vi "Station Detail Main.vi"(8 "error in (no error)":errorcluster, 11 "AI in":refnum<class "AI.lvclass">) -> (0 "error out":errorcluster, 2 "Station Out":T1=enum."ImformOut", 3 "AI out":refnum<class "AI.lvclass">)   [LabVIEW 2019, in "AI.lvclass"]
uses:
  AI.lvclass
  Ctrl/Station Action.ctl
  Ctrl/ProjectStepSelect.ctl
  Ctrl/StationCmdSelect.ctl
  Ctrl/Auto Inspection Station Name2.ctl
  Ctrl/Auto Inspection Data Name.ctl
  Ctrl/S2 Station IO.ctl
  Ctrl/MeasureDisplayTab.ctl
  Ctrl/Table Save.ctl
  Ctrl/S2 Station Input.ctl
  Global/Process Global.vi
  LLB/Commonly VI/Main Glb.vi
  LineScan/LineScan.lvclass
  LLB/Commonly VI.lvlib
panel:
  out "ToolStringOut_P1_2 2":string
  out "P1 Receive 2":string[](array[string])
  out "ToolStringOut_P1 2":string
  out "Program receive 2":string
  out "Initial receive 2":string
  out "Array":string[](array[string])
  out "Blue Scan receive":string
  out "S1 ChkSum":string
  out "S1 ToolStringOut":string
  out "ToolStringOut_P1_2":string
  out "P1 Receive":string[](array[string])
  out "ToolStringOut_P1":string
  out "ToolStringOut_Init":string
  out "Initial_ChkSum":string
  in  "Table Control":string[][](table)=[["PCBA BARCODE", ""], ["硬體(Tool初始化)", ""], ["company(Tool初始化)", ""], ["耗電流 uA(電流表)", "T"], ["電池負載電壓", "T"], ["晶片ID(Tool FORMAT)", "F"], ["雷雕ID(TOOl scan、藍芽接收器)", "S"], ["Format(Tool FORMAT)", "F"], ["Programe(Tool Programe)", "P"]]
  out "Numeric":dbl
  out "subarray":string[](array[string])
  out "T2 buffer":string
  out "T2 μA":dbl format="%#_6f"
  out "T1 buffer":string
  out "T1 μA":dbl format="%#_6f"
  out "S2 receive":string
  out "Blue Scan2 receive":string
  out "S1 receive":string
  out "Program receive":string
  out "format receive":string
  out "Initial receive":string
  out "present":i32
  out "Retry":i32
  out "Act Step":i32
  out "retry次數":string[](array[string])
  out "CurrentCmd":string
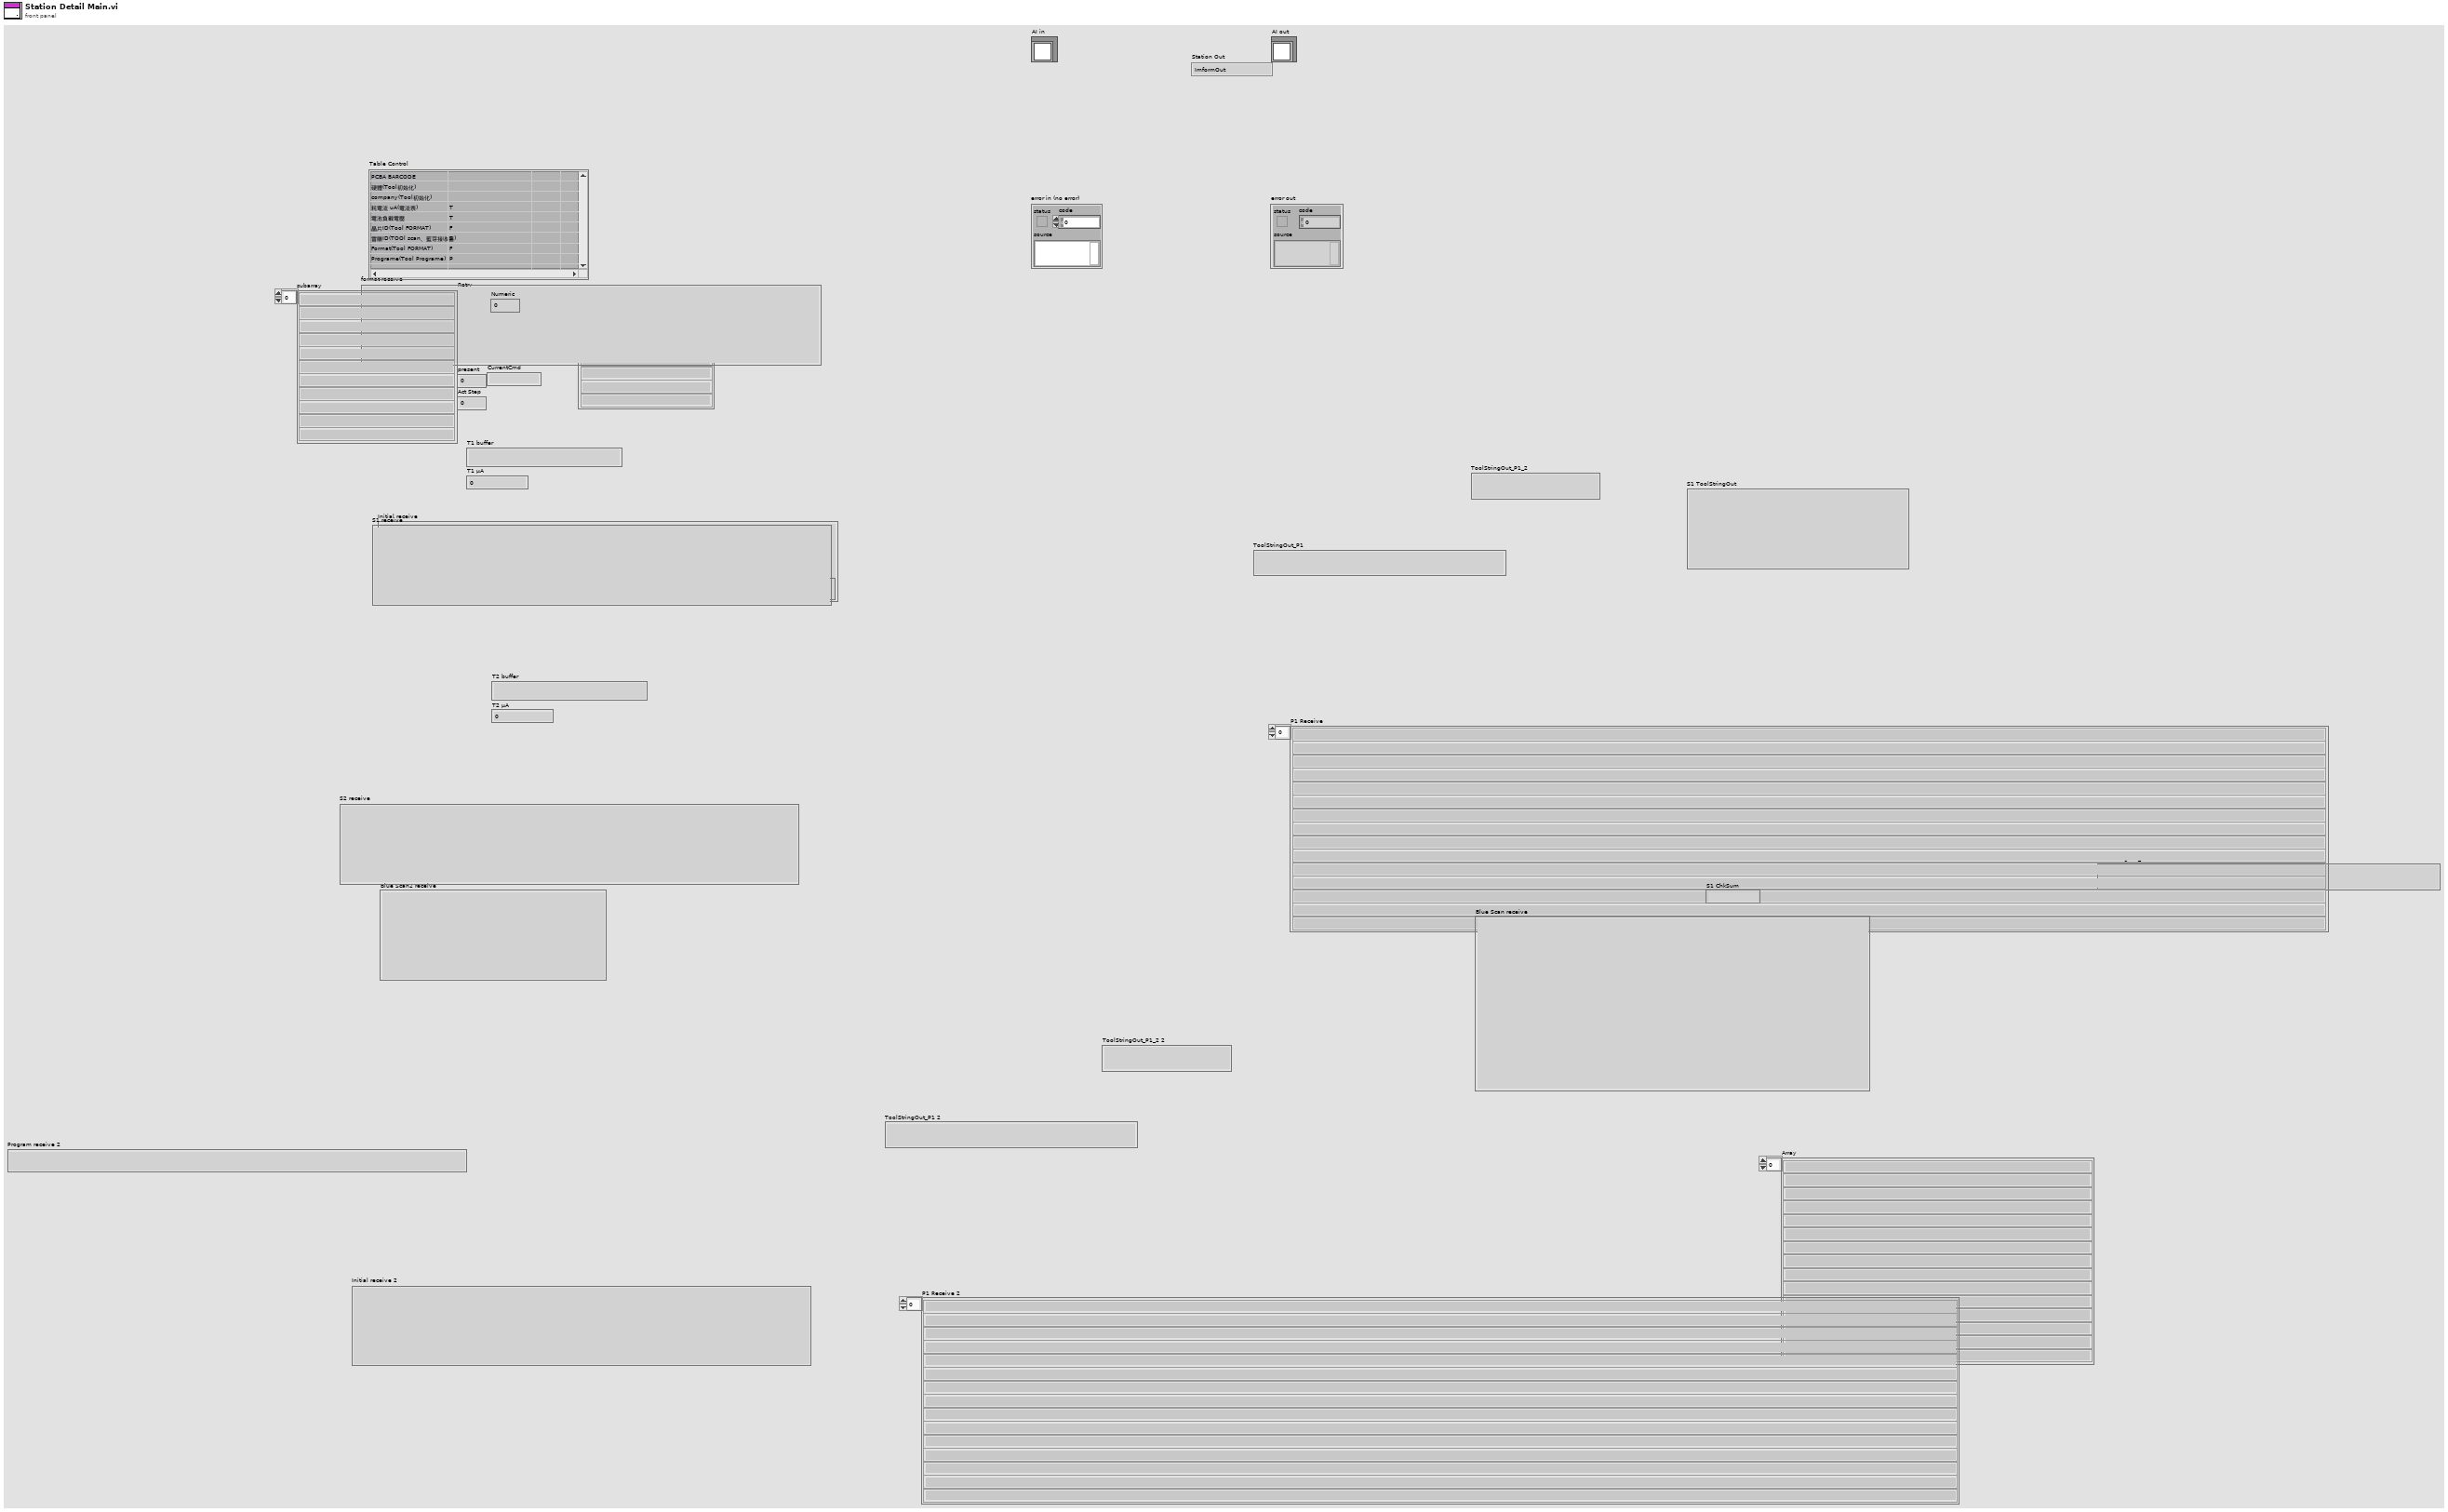
[diagram p1: front panel]
types:
  T1 = typedef "Station Action.ctl" = enum16{"Wait Item In", "Dectect Action", "ImformOut"}
  T2 = typedef "StationCmdSelect.ctl" = enum16{"Action", "Command", "Return", "DTime", "Retry"}
  T3 = typedef "Auto Inspection Data Name.ctl" = enum16{"LocalRun", "ItemSN(TimeCode)", "CurrentAction", "Error", "Data", "OKNG", "電壓值", "電壓值判斷", "電流值", "電流值判斷", "Laser1 Data", "Laser2 Data", "Laser OKNG", "StationNO"}
  T4 = typedef "Auto Inspection Station Name2.ctl" = enum16{"S1Barcode", "S2Measure", "S3Measure", "S4Measure", "S5Measure", "S11_LaserCheck", "S8_Vision AI"}
  T5 = typedef "Table Save.ctl" = enum16{"initial", "Add", "Write", "Replace", "Delete", "REad", "RedTable", "Load"}
  T6 = typedef "MeasureDisplayTab.ctl" = enum16{"Tray Barcode", "PCBA BARCODE", "硬體(Tool初始化)", "company(Tool初始化)", "耗電流 uA(電流表)", "電池負載電壓", "晶片ID(Tool FORMAT)", "雷雕ID(TOOl scan、藍芽接收器)", "Format(Tool FORMAT)", "Programe(Tool Programe)", "MAC(藍芽接收器)", "ID(藍芽接收器)", "KPA(藍芽接收器)", "溫度(藍芽接收器)", "SENSOR電池電壓(藍芽接收器)", "RSSI(藍芽接收器)", "SensorType_315(FSK scan)", "FSKsnVol_315(FSK scan)", "FSKscanl_315(FSK scan)", "P_315(FSK scan)", "T_315(FSK scan)", "SensorType_433(ASK scan)", "ASKsnVol_433(ASK scan)", "ASKscan_433(ASK scan)", "P_433(ASK scan)", "T_433(ASK scan)", "測高Data"}
  T7 = typedef "S2 Station Input.ctl" = enum16{"00PLC Alive clock", "01PLC狀態(手動)", "02PLC狀態(自動)", "03PLC Alarm", "04備用", "05備用", "06備用", "07備用", "08備用", "09備用", "10載盤有料for條碼", "11_備用", "12_備用", "13_備用", "14_備用", "15_備用", "16_備用", "17_備用", "18_備用", "19_備用", "20_載盤有料訊號ForS2站", "21_PLC下達可測電流訊號", "22_PLC下達可測電壓訊號"}
  T8 = typedef "ProjectStepSelect.ctl" = enum16{"ProjectName", "Name", "Initial", "Reset", "Format", "Program1", "Program2", "Scan", "Finish", "MToolWork", "DataCheck", "DataSave", "OutputPLC", "WaitInputS1", "WaitInputOff"}
  T9 = typedef "S2 Station IO.ctl" = enum16{"S2站PC動作中_20", "電流量測完成產品OK_21", "電流量測完成產品NG_22", "S2站Format 執行_23", "S2 Format OK_24", "S2 Format NG_25", "S2站燒入執行_26", "S2站燒入OK_27", "S2站燒入NG_28", "S2站動作完成_29", "S3 PC動作中_30", "S3 Format 此站執行_31", "S3 Format OK_32", "S3 Format NG_33", "S3 燒入程式 此站執行_34", "S3 燒入程式 OK_35", "S3 燒入程式 NG_36", "S3 備用_37", "S3 備用_38", "S3 動作完成_39", "S4 PC動作中_40", "S4 量測完成 產品正常_41", "S4 量測完成 產品NG_42", "S4 Format 此站執行_43", "S4 Format OK_44", "S4 Format NG_45", "S4 燒入 此站不執行_46", "S4 燒入程式 OK_47", "S4 燒入程式 NG_48", "S4 藍芽Scan OK_49", "S4 藍芽Scan NG_50", "S4 動作完成_51", "給PLC要量電流訊號", "給PLC要量電壓訊號"}
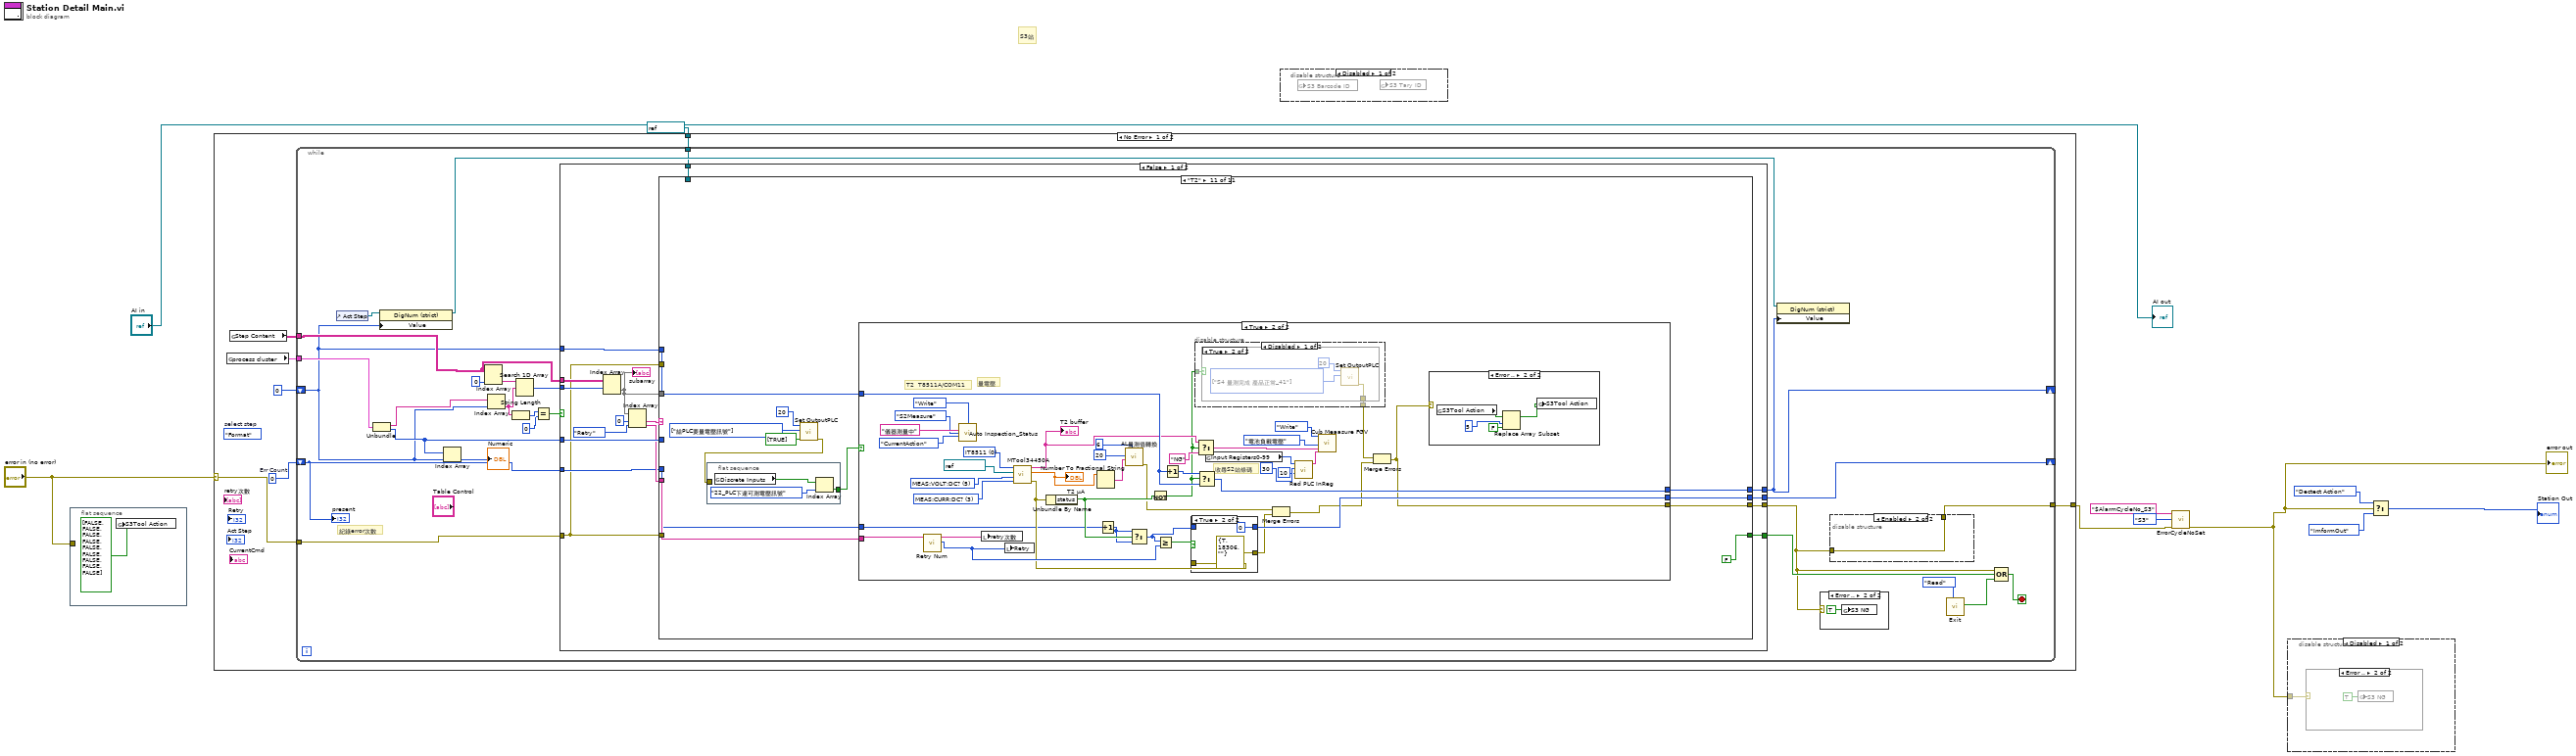
[diagram p0: block diagram]
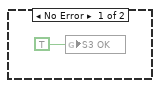
[diagram p2: hidden frame]
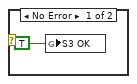
[diagram p5: hidden frame]
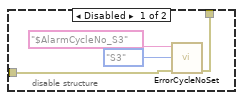
[diagram p6: hidden frame]
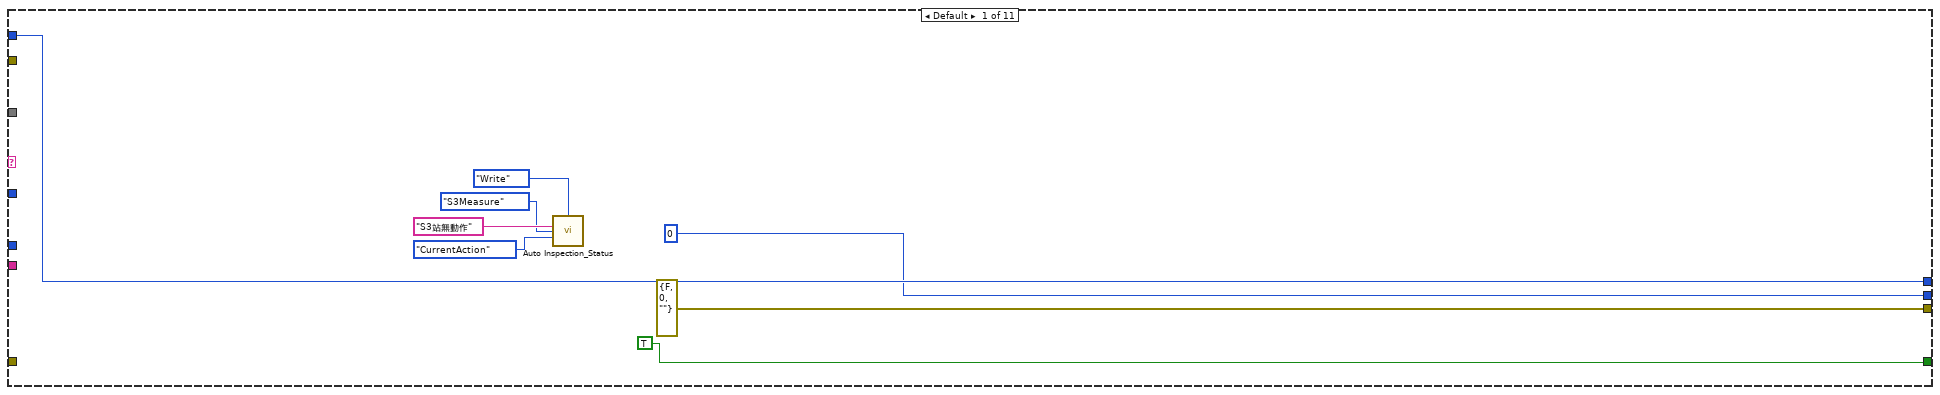
[diagram p7: hidden frame]
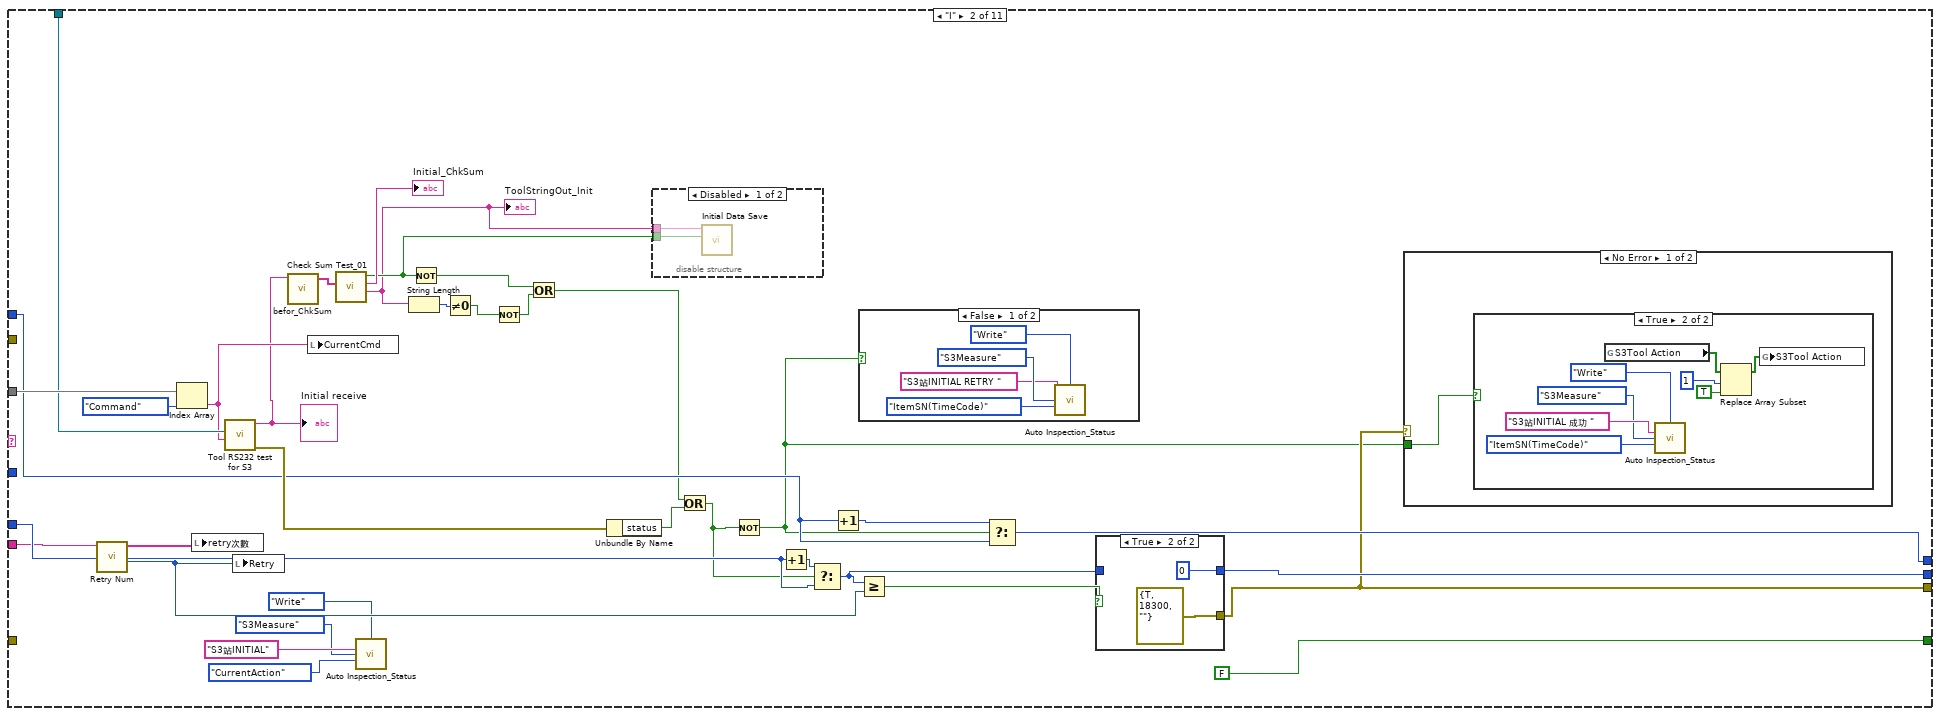
[diagram p8: hidden frame]
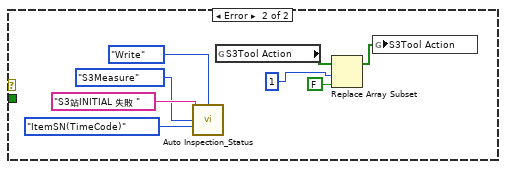
[diagram p12: hidden frame]
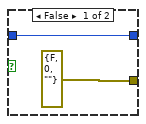
[diagram p13: hidden frame]
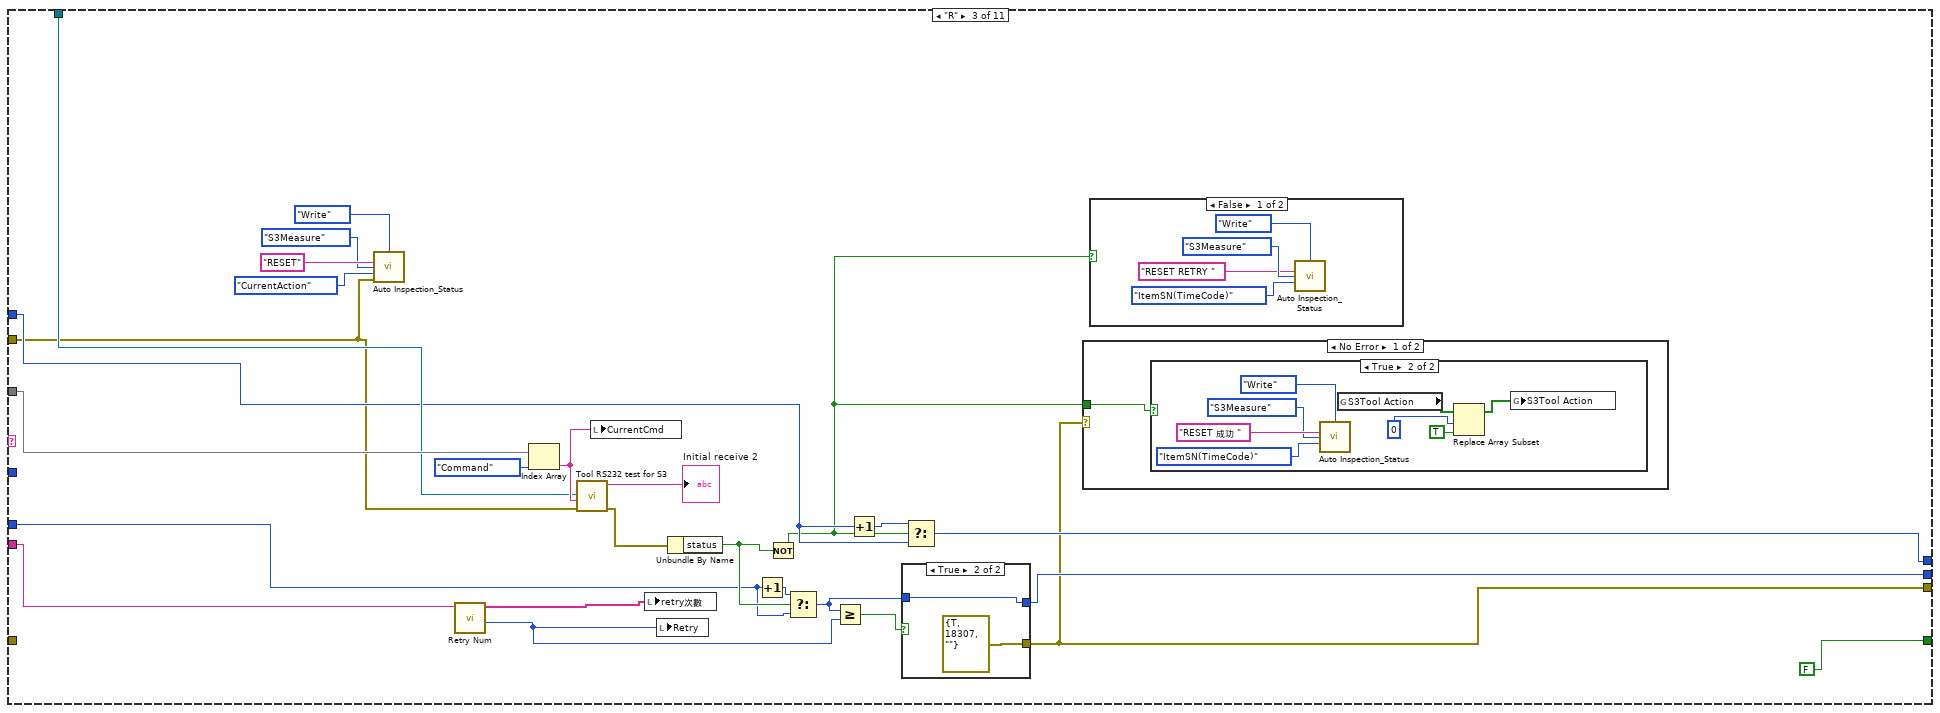
[diagram p14: hidden frame]
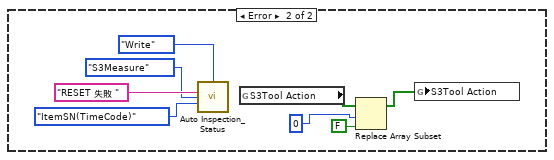
[diagram p17: hidden frame]
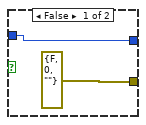
[diagram p18: hidden frame]
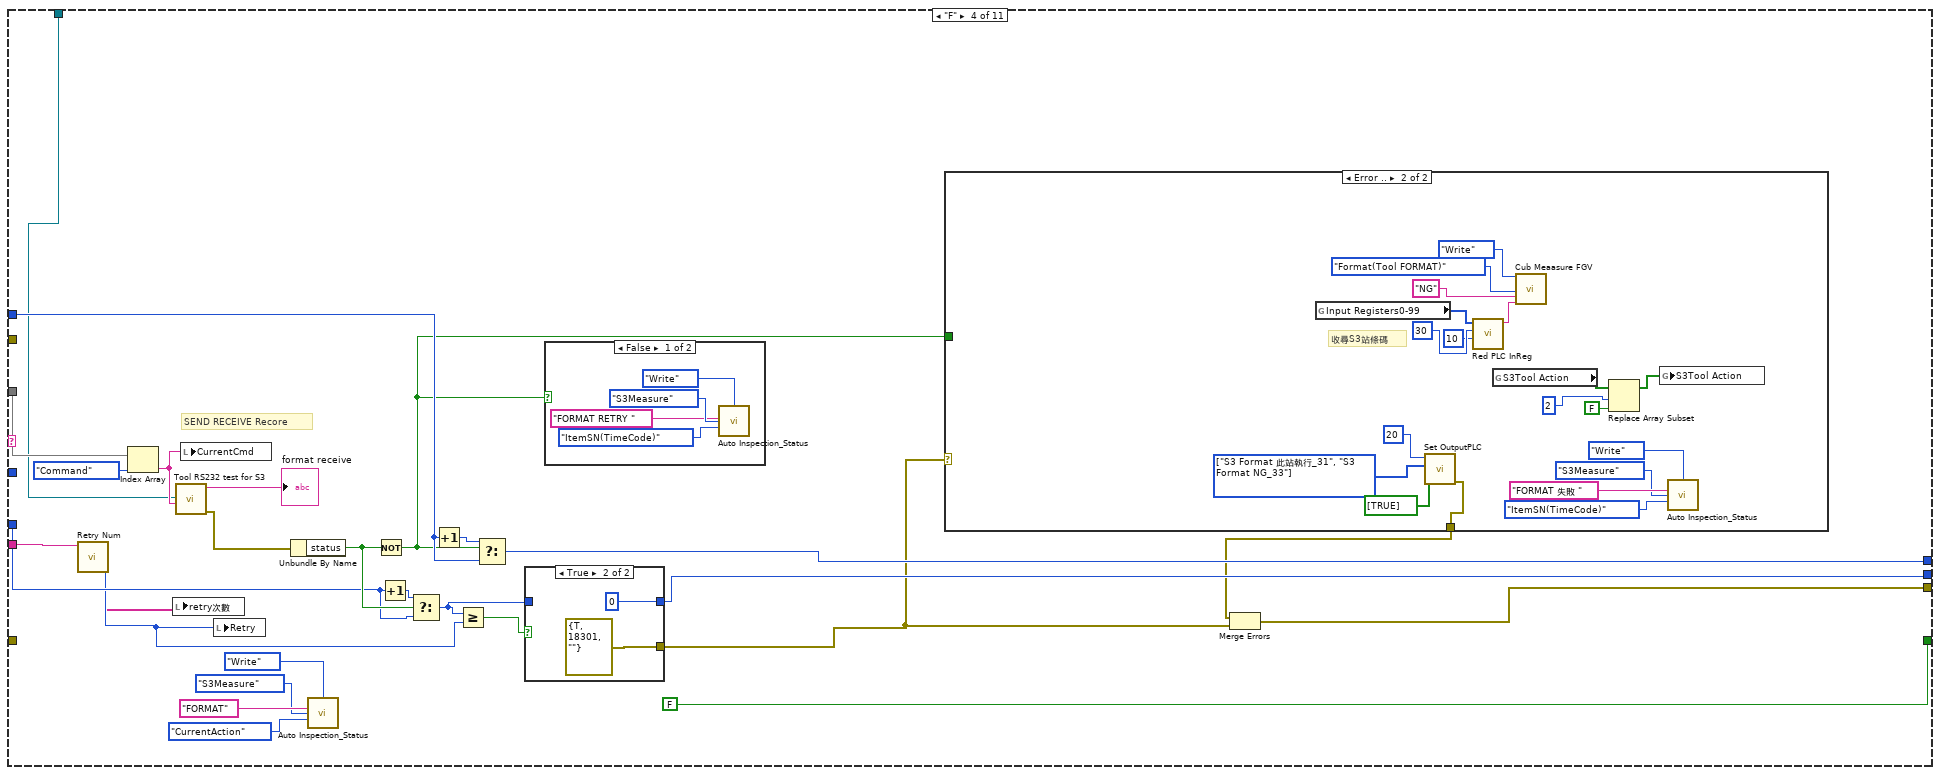
[diagram p19: hidden frame]
diagram:
  # "S3站"
  n1 = flat-sequence {
    tunnel: "error in (no error)" -> [_]
    frame #0 {
      n2 = global write "Process Global.vi" "S3Tool Action"(bool[] [FALSE, FALSE, FALSE, FALSE, FALSE, FALSE, FALSE, FALSE, FALSE] ("S3Tool Action")) -> ()
    }
  }
  n3 = case shown="No Error" "error in (no error)" {
    selector: "error in (no error)" -> [w13 w752]
    tunnel: [w18 w752] -> w2
    tunnel: refnum<visa-resource-name> "COM2" ("VISA resource name") -> [w12 _]
    frame No Error {
      w14 = 0  # Err Count
      (unwired) ProjectStepSelect."Format"  # select step
      n4 = global read "Process Global.vi" "process cluster"() -> (w16:cluster{string[], i32[]})
      n5 = global read "Process Global.vi" "Step Content"() -> (w17:string[][])
      n6 = while {
        tunnel: [w20] -> w18
        shift-right: [w26] -> _
        shift-left: 0 -> [w27]
        shift-right: [w29] -> _
        shift-left: w14 -> [w30]
        tunnel: w17 -> [w41]
        tunnel: w16 -> [w40]
        tunnel: w13 -> [w24]
        tunnel: w12 -> [w23]
        stop <- w42 stop-if-true
        # "紀錄error次數"
        n7 = control-ref of="Act Step"() -> (w28:refnum<vi>)
        n8 = Unbundle(w40) -> (w43:string[], w44:i32[])
        n9 = property class="DigNum (strict)"(reference=w28, "Value"=w27) -> (reference out=w25:refnum<vi>)  [unwired: 1 in, 1 out]
        n10 = Index Array(array=w44, index=w27) -> (element=→"Numeric":i32)
        n11 = Index Array(array=w41, index (col)=0 ("disabled index (col)")) -> (element=w38:string[])  [unwired: 1 in]
        n12 = Index Array(array=w43, index=w27) -> (element=w34:string)
        n13 = String Length(string=w34) -> (length=w35:i32)
        n14 = Search 1D Array(1D array=w38, element=w34) -> (index of element=w37:i32)  [unwired: 1 in]
        n15 = Equal?(x=w35, y=0) -> (x = y?=w32:bool)
        n16 = case shown="False" w32 {
          tunnel: w44 -> [w67 _]
          tunnel: w41 -> [w66 _]
          tunnel: w37 -> [w65 _]
          tunnel: [w54 TRUE] -> w31
          tunnel: [w57 errorcluster {"status"=FALSE, "code"=0, "source"=""} ("error constant")] -> w19
          tunnel: w27 -> [w60 _]
          tunnel: [w59 0] -> w26
          tunnel: w30 -> [w58 _]
          tunnel: [w56 0 ("Err Count")] -> w29
          tunnel: w24 -> [w53 _]
          tunnel: w23 -> [w52 _]
          frame False {
            n17 = Index Array(array=w66, index (row)=w65) -> (element=w61:string[])  [unwired: 1 in]
            "subarray" <- w61
            n18 = Index Array(array=w61, index #1=0 ("index"), index #2=StationCmdSelect."Retry") -> (element #1=w63:string, element #2=w62:string)
            n19 = case shown="\"T2\"" w63 {
              tunnel: w67 -> [_ _ _ _ _ _ _ _ w580 _ _]
              tunnel: w62 -> [_ w100 w147 w215 w317 w374 w498 w552 _ w591 w672]
              tunnel: w61 -> [_ w102 w151 w214 w319 w375 w497 w553 _ _ _]
              tunnel: w60 -> [w75 w91 w148 w210 w318 w371 w496 w555 w575 w589 w674]
              tunnel: [w75 w98 w143 w212 w314 w372 w500 w550 w574 w588 w673] -> w59
              tunnel: w58 -> [_ w101 w146 w206 w316 w373 w495 w551 _ w592 w671]
              tunnel: [errorcluster {"status"=FALSE, "code"=0, "source"=""} ("error constant") w77 w140 w196 w274 w368 w493 w548 errorcluster {"status"=FALSE, "code"=0, "source"=""} ("error constant") w587 w670] -> w57
              tunnel: [0 ("Err Count") w99 w142 w201 w315 w369 w499 w549 0 ("Err Count") w590 w675] -> w56
              tunnel: [TRUE FALSE FALSE FALSE FALSE FALSE FALSE FALSE FALSE FALSE FALSE] -> w54
              tunnel: w53 -> [_ _ _ _ _ _ _ _ _ _ _]
              tunnel: w53 -> [_ _ w139 _ w273 w364 w452 w554 _ _ _]
              tunnel: w52 -> [_ w92 w149 w191 w282 w376 w465 w513 _ _ _]
              frame Default {
                n20 = call "Auto Inspection_Status.vi"("Action"=enum16{"Initial", "Write", "Read"}."Write", "DataIn"="S3站無動作", "Station"=Auto_Inspection_Station_Name2."S3Measure", "Data"=Auto_Inspection_Data_Name."CurrentAction") -> ()  [unwired: 9 in, 3 out]
              }
              frame "I" {
                n21 = call "Retry Num.vi"("String"=w100) -> ("Numeric"=w107:i32, "retry次數"=w104:string[])  [unwired: 9 in]
                n22 = Index Array(array=w102, index=StationCmdSelect."Command") -> (element=w84:string)
                n23 = local write "retry次數"(w104) -> ()
                n24 = call "Tool RS232 test for S3.vi"("Cmd In"=w84, "VISA resource name"=w92) -> ("error out"=w110:errorcluster, "receive string"=w78:string)  [unwired: 8 in]
                "Initial receive" <- w78
                n25 = local write "Retry"(w107) -> ()
                n26 = call "befor_ChkSum.vi"("ToolString Input"=w78) -> ("Array"=w89:string[])  [unwired: 9 in, 1 out]
                n27 = local write "CurrentCmd"(w84) -> ()
                n28 = call "Check Sum Test_01.vi"("Array"=w89) -> ("ToolStringOut_01"=w79:string, "ChkSum"=→"Initial_ChkSum":string, "x = y?"=w80:bool)  [unwired: 8 in]
                "ToolStringOut_Init" <- w79
                n29 = call "Auto Inspection_Status.vi"("Action"=enum16{"Initial", "Write", "Read"}."Write", "DataIn"="S3站INITIAL", "Station"=Auto_Inspection_Station_Name2."S3Measure", "Data"=Auto_Inspection_Data_Name."CurrentAction") -> ()  [unwired: 9 in, 3 out]
                n30 = String Length(string=w79) -> (length=w86:i32)
                n31 = Not(x=w80) -> (.not. x?=w88:bool)
                n32 = Not Equal To 0?(x=w86) -> (x != 0?=w85:bool)
                n33 = Not(x=w85) -> (.not. x?=w87:bool)
                n34 = Or(x=w88, y=w87) -> (x .or. y?=w83:bool)
                n35 = Unbundle By Name(w110) -> ("status"=w82:bool)
                n36 = disable-structure shown="Disabled" {
                  disable-tunnel: w80 -> [w116 _]
                  disable-tunnel: w79 -> [w115 _]
                  frame Disabled {
                    n37 = call "Initial Data Save.vi"("OK and NG"=w116, "String In"=w115) -> ()  [unwired: 9 in, 1 out]
                  }
                  frame Enabled {
                  }
                }
                n38 = Or(x=w83, y=w82) -> (x .or. y?=w81:bool)
                n39 = Not(x=w81) -> (.not. x?=w76:bool)
                n40 = Increment(x=w101) -> (x+1=w108:i32)
                n41 = Select(t=w108, s=w81, f=w101) -> (s? t:f=w105:i32)
                n42 = Increment(x=w91) -> (x+1=w109:i32)
                n43 = case shown="False" w76 {
                  frame False {
                    n44 = call "Auto Inspection_Status.vi"("Action"=enum16{"Initial", "Write", "Read"}."Write", "DataIn"="S3站INITIAL RETRY ", "Station"=Auto_Inspection_Station_Name2."S3Measure", "Data"=Auto_Inspection_Data_Name."ItemSN(TimeCode)") -> ()  [unwired: 9 in, 3 out]
                  }
                  frame True {
                  }
                }
                n45 = Greater Or Equal?(x=w105, y=w107) -> (x >= y?=w106:bool)
                n46 = Select(t=w109, s=w76, f=w91) -> (s? t:f=w98:i32)
                n47 = case shown="True" w106 {
                  tunnel: [errorcluster {"status"=FALSE, "code"=0, "source"=""} ("error constant") errorcluster {"status"=TRUE, "code"=18300, "source"=""} ("error constant")] -> w77
                  tunnel: w105 -> [w134 _]
                  tunnel: [w134 0] -> w99
                  frame False {
                  }
                  frame True {
                  }
                }
                n48 = case shown="No Error" w77 {
                  tunnel: w76 -> [w117 _]
                  frame No Error {
                    n49 = case shown="True" w117 {
                      frame False {
                      }
                      frame True {
                        n50 = global read "Process Global.vi" "S3Tool Action"() -> (w121:bool[])
                        n51 = call "Auto Inspection_Status.vi"("Action"=enum16{"Initial", "Write", "Read"}."Write", "DataIn"="S3站INITIAL 成功 ", "Station"=Auto_Inspection_Station_Name2."S3Measure", "Data"=Auto_Inspection_Data_Name."ItemSN(TimeCode)") -> ()  [unwired: 9 in, 3 out]
                        n52 = Replace Array Subset(array=w121, new element=TRUE ("new element/subarray"), index=1) -> (w118:bool[])
                        n53 = global write "Process Global.vi" "S3Tool Action"(w118) -> ()
                      }
                    }
                  }
                  frame Error {
                    n54 = call "Auto Inspection_Status.vi"("Action"=enum16{"Initial", "Write", "Read"}."Write", "DataIn"="S3站INITIAL 失敗 ", "Station"=Auto_Inspection_Station_Name2."S3Measure", "Data"=Auto_Inspection_Data_Name."ItemSN(TimeCode)") -> ()  [unwired: 9 in, 3 out]
                    n55 = global read "Process Global.vi" "S3Tool Action"() -> (w129:bool[])
                    n56 = Replace Array Subset(array=w129, new element=FALSE ("new element/subarray"), index=1) -> (w126:bool[])
                    n57 = global write "Process Global.vi" "S3Tool Action"(w126) -> ()
                  }
                }
              }
              frame "R" {
                n58 = call "Auto Inspection_Status.vi"("Action"=enum16{"Initial", "Write", "Read"}."Write", "DataIn"="RESET", "Station"=Auto_Inspection_Station_Name2."S3Measure", "Data"=Auto_Inspection_Data_Name."CurrentAction", "error in"=w139) -> ()  [unwired: 8 in, 3 out]
                n59 = call "Retry Num.vi"("String"=w147) -> ("Numeric"=w144:i32, "retry次數"=w145:string[])  [unwired: 9 in]
                n60 = Index Array(array=w151, index=StationCmdSelect."Command") -> (element=w150:string)
                n61 = call "Tool RS232 test for S3.vi"("error in (no error)"=w139, "Cmd In"=w150, "VISA resource name"=w149) -> ("error out"=w158:errorcluster, "receive string"=→"Initial receive 2":string)  [unwired: 7 in]
                n62 = local write "CurrentCmd"(w150) -> ()
                n63 = local write "retry次數"(w145) -> ()
                n64 = local write "Retry"(w144) -> ()
                n65 = Unbundle By Name(w158) -> ("status"=w160:bool)
                n66 = Increment(x=w146) -> (x+1=w161:i32)
                n67 = Not(x=w160) -> (.not. x?=w138:bool)
                n68 = Select(t=w161, s=w160, f=w146) -> (s? t:f=w162:i32)
                n69 = Greater Or Equal?(x=w162, y=w144) -> (x >= y?=w163:bool)
                n70 = Increment(x=w148) -> (x+1=w159:i32)
                n71 = case shown="True" w163 {
                  tunnel: [errorcluster {"status"=FALSE, "code"=0, "source"=""} ("error constant") errorcluster {"status"=TRUE, "code"=18307, "source"=""} ("error constant")] -> w140
                  tunnel: w162 -> [w185 w187]
                  tunnel: [w185 w187] -> w142
                  frame False {
                  }
                  frame True {
                  }
                }
                n72 = Select(t=w159, s=w138, f=w148) -> (s? t:f=w143:i32)
                n73 = case shown="No Error" w140 {
                  tunnel: w138 -> [w168 _]
                  frame No Error {
                    n74 = case shown="True" w168 {
                      frame False {
                      }
                      frame True {
                        n75 = call "Auto Inspection_Status.vi"("Action"=enum16{"Initial", "Write", "Read"}."Write", "DataIn"="RESET 成功 ", "Station"=Auto_Inspection_Station_Name2."S3Measure", "Data"=Auto_Inspection_Data_Name."ItemSN(TimeCode)") -> ()  [unwired: 9 in, 3 out]
                        n76 = global read "Process Global.vi" "S3Tool Action"() -> (w172:bool[])
                        n77 = Replace Array Subset(array=w172, new element=TRUE ("new element/subarray"), index=0) -> (w169:bool[])
                        n78 = global write "Process Global.vi" "S3Tool Action"(w169) -> ()
                      }
                    }
                  }
                  frame Error {
                    n79 = call "Auto Inspection_Status.vi"("Action"=enum16{"Initial", "Write", "Read"}."Write", "DataIn"="RESET 失敗 ", "Station"=Auto_Inspection_Station_Name2."S3Measure", "Data"=Auto_Inspection_Data_Name."ItemSN(TimeCode)") -> ()  [unwired: 9 in, 3 out]
                    n80 = global read "Process Global.vi" "S3Tool Action"() -> (w180:bool[])
                    n81 = Replace Array Subset(array=w180, new element=FALSE ("new element/subarray"), index=0) -> (w177:bool[])
                    n82 = global write "Process Global.vi" "S3Tool Action"(w177) -> ()
                  }
                }
                n83 = case shown="False" w138 {
                  frame False {
                    n84 = call "Auto Inspection_Status.vi"("Action"=enum16{"Initial", "Write", "Read"}."Write", "DataIn"="RESET RETRY ", "Station"=Auto_Inspection_Station_Name2."S3Measure", "Data"=Auto_Inspection_Data_Name."ItemSN(TimeCode)") -> ()  [unwired: 9 in, 3 out]
                  }
                  frame True {
                  }
                }
              }
              frame "F" {
                # "SEND RECEIVE Recore"
                n85 = call "Retry Num.vi"("String"=w215) -> ("Numeric"=w205:i32, "retry次數"=w200:string[])  [unwired: 9 in]
                n86 = Index Array(array=w214, index=StationCmdSelect."Command") -> (element=w199:string)
                n87 = local write "retry次數"(w200) -> ()
                n88 = call "Tool RS232 test for S3.vi"("Cmd In"=w199, "VISA resource name"=w191) -> ("error out"=w211:errorcluster, "receive string"=→"format receive":string)  [unwired: 8 in]
                n89 = local write "CurrentCmd"(w199) -> ()
                n90 = local write "Retry"(w205) -> ()
                n91 = Unbundle By Name(w211) -> ("status"=w208:bool)
                n92 = call "Auto Inspection_Status.vi"("Action"=enum16{"Initial", "Write", "Read"}."Write", "DataIn"="FORMAT", "Station"=Auto_Inspection_Station_Name2."S3Measure", "Data"=Auto_Inspection_Data_Name."CurrentAction") -> ()  [unwired: 9 in, 3 out]
                n93 = Not(x=w208) -> (.not. x?=w189:bool)
                n94 = Increment(x=w206) -> (x+1=w207:i32)
                n95 = Select(t=w207, s=w208, f=w206) -> (s? t:f=w202:i32)
                n96 = Increment(x=w210) -> (x+1=w209:i32)
                n97 = Greater Or Equal?(x=w202, y=w205) -> (x >= y?=w204:bool)
                n98 = Select(t=w209, s=w189, f=w210) -> (s? t:f=w212:i32)
                n99 = case shown="True" w204 {
                  tunnel: [errorcluster {"status"=FALSE, "code"=0, "source"=""} ("error constant") errorcluster {"status"=TRUE, "code"=18301, "source"=""} ("error constant")] -> w190
                  tunnel: w202 -> [w264 _]
                  tunnel: [w264 0] -> w201
                  frame False {
                  }
                  frame True {
                  }
                }
                n100 = case shown="False" w189 {
                  frame False {
                    n101 = call "Auto Inspection_Status.vi"("Action"=enum16{"Initial", "Write", "Read"}."Write", "DataIn"="FORMAT RETRY ", "Station"=Auto_Inspection_Station_Name2."S3Measure", "Data"=Auto_Inspection_Data_Name."ItemSN(TimeCode)") -> ()  [unwired: 9 in, 3 out]
                  }
                  frame True {
                  }
                }
                n102 = case shown="Error .." w190 {
                  tunnel: [w221 w261] -> w197
                  tunnel: w189 -> [w220 _]
                  frame No Error {
                    n103 = case shown="True" w220 {
                      tunnel: [_ w242] -> w221
                      frame False {
                      }
                      frame True {
                        w243 = T9[] [enum."S3 Format 此站執行_31", enum."S3 Format OK_32"] items=["S2站PC動作中_20", "電流量測完成產品OK_21", "電流量測完成產品NG_22", "S2站Format 執行_23", "S2 Format OK_24", "S2 Format NG_25", "S2站燒入執行_26", "S2站燒入OK_27", "S2站燒入NG_28", "S2站動作完成_29", "S3 PC動作中_30", "S3 Format 此站執行_31", "S3 Format OK_32", "S3 Format NG_33", "S3 燒入程式 此站執行_34", "S3 燒入程式 OK_35", "S3 燒入程式 NG_36", "S3 備用_37", "S3 備用_38", "S3 動作完成_39", "S4 PC動作中_40", "S4 量測完成 產品正常_41", "S4 量測完成 產品NG_42", "S4 Format 此站執行_43", "S4 Format OK_44", "S4 Format NG_45", "S4 燒入 此站不執行_46", "S4 燒入程式 OK_47", "S4 燒入程式 NG_48", "S4 藍芽Scan OK_49", "S4 藍芽Scan NG_50", "S4 動作完成_51", "給PLC要量電流訊號", "給PLC要量電壓訊號"]
                        # "收尋S3站條碼"
                        n104 = global read "Main Glb.vi" "Input Registers0-99"() -> (w232:u16[])
                        n105 = call "Red PLC InReg.vi"("length"=10, "index"=30, "Input Registers Arr"=w232) -> ("Rad In Reg"=w225:string)  [unwired: 7 in, 1 out]
                        n106 = call "Cub Meaasure FGV.vi"("Action"=Table_Save."Write" ("Enum"), "Save Index"=MeasureDisplayTab."Format(Tool FORMAT)", "DataIn"="OK", "SN"=w225) -> ("error out"=w224:errorcluster)  [unwired: 8 in, 7 out]
                        n107 = global write "Main Glb.vi" "S3 Barcode ID"(w225) -> ()
                        n108 = call "Cub Meaasure FGV.vi"("Action"=Table_Save."REad" ("Enum"), "Save Index"=MeasureDisplayTab."Tray Barcode", "SN"=w225, "error in (no error)"=w224) -> ("Read Index Data"=w223:string)  [unwired: 8 in, 7 out]
                        n109 = call "Set OutputPLC.vi"("Address In"=20, "Array 2"=w243, "Sat Coils"=bool[] [TRUE]) -> ("Error Out"=w242:errorcluster[])  [unwired: 7 in]
                        n110 = global write "Main Glb.vi" "S3 Tary ID"(w223) -> ()
                        n111 = global read "Process Global.vi" "S3Tool Action"() -> (w235:bool[])
                        n112 = Replace Array Subset(array=w235, new element=TRUE ("new element/subarray"), index=2) -> (w228:bool[])
                        n113 = call "Auto Inspection_Status.vi"("Action"=enum16{"Initial", "Write", "Read"}."Write", "DataIn"="FORMAT完成", "Station"=Auto_Inspection_Station_Name2."S3Measure", "Data"=Auto_Inspection_Data_Name."ItemSN(TimeCode)") -> ()  [unwired: 9 in, 3 out]
                        n114 = global write "Process Global.vi" "S3Tool Action"(w228) -> ()
                      }
                    }
                  }
                  frame Error {
                    w263 = T9[] [enum."S3 Format 此站執行_31", enum."S3 Format NG_33"] items=["S2站PC動作中_20", "電流量測完成產品OK_21", "電流量測完成產品NG_22", "S2站Format 執行_23", "S2 Format OK_24", "S2 Format NG_25", "S2站燒入執行_26", "S2站燒入OK_27", "S2站燒入NG_28", "S2站動作完成_29", "S3 PC動作中_30", "S3 Format 此站執行_31", "S3 Format OK_32", "S3 Format NG_33", "S3 燒入程式 此站執行_34", "S3 燒入程式 OK_35", "S3 燒入程式 NG_36", "S3 備用_37", "S3 備用_38", "S3 動作完成_39", "S4 PC動作中_40", "S4 量測完成 產品正常_41", "S4 量測完成 產品NG_42", "S4 Format 此站執行_43", "S4 Format OK_44", "S4 Format NG_45", "S4 燒入 此站不執行_46", "S4 燒入程式 OK_47", "S4 燒入程式 NG_48", "S4 藍芽Scan OK_49", "S4 藍芽Scan NG_50", "S4 動作完成_51", "給PLC要量電流訊號", "給PLC要量電壓訊號"]
                    # "收尋S3站條碼"
                    n115 = global read "Main Glb.vi" "Input Registers0-99"() -> (w250:u16[])
                    n116 = call "Set OutputPLC.vi"("Address In"=20, "Array 2"=w263, "Sat Coils"=bool[] [TRUE]) -> ("Error Out"=w261:errorcluster[])  [unwired: 7 in]
                    n117 = call "Red PLC InReg.vi"("length"=10, "index"=30, "Input Registers Arr"=w250) -> ("Rad In Reg"=w253:string)  [unwired: 7 in, 1 out]
                    n118 = global read "Process Global.vi" "S3Tool Action"() -> (w256:bool[])
                    n119 = call "Cub Meaasure FGV.vi"("Action"=Table_Save."Write" ("Enum"), "Save Index"=MeasureDisplayTab."Format(Tool FORMAT)", "DataIn"="NG", "SN"=w253) -> ()  [unwired: 8 in, 8 out]
                    n120 = Replace Array Subset(array=w256, new element=FALSE ("new element/subarray"), index=2) -> (w246:bool[])
                    n121 = global write "Process Global.vi" "S3Tool Action"(w246) -> ()
                    n122 = call "Auto Inspection_Status.vi"("Action"=enum16{"Initial", "Write", "Read"}."Write", "DataIn"="FORMAT 失敗 ", "Station"=Auto_Inspection_Station_Name2."S3Measure", "Data"=Auto_Inspection_Data_Name."ItemSN(TimeCode)") -> ()  [unwired: 9 in, 3 out]
                  }
                }
                n123 = Merge Errors(w197, w190) -> (w196:errorcluster)
              }
              frame "P1" {
                # "經過燒錄後第二次Tool回傳"
                # "下Cmd後第一次Tool回傳"
                # "收尋S3站條碼"
                # "SEND RECEIVE Recore"
                n124 = Index Array(array=w319, index=StationCmdSelect."Command") -> (element=w283:string)
                n125 = call "Tool RS232 test for S3.vi"("error in (no error)"=w273, "Cmd In"=w283, "VISA resource name"=w282) -> ("error out"=w280:errorcluster, "receive string"=→"Program receive":string)  [unwired: 7 in]
                n126 = local write "CurrentCmd"(w283) -> ()
                n127 = call "befor_ChkSum.vi"("ToolString Input"=w283) -> ("Array"=w300:string[])  [unwired: 9 in, 1 out]
                n128 = call "Auto Inspection_Status.vi"("Action"=enum16{"Initial", "Write", "Read"}."Write", "DataIn"="PROGRAM1", "Station"=Auto_Inspection_Station_Name2."S3Measure", "Data"=Auto_Inspection_Data_Name."CurrentAction", "error in"=w273) -> ()  [unwired: 8 in, 3 out]
                n129 = call "Check Sum Test_01.vi"("Array"=w300) -> ("ToolStringOut_01"=w297:string, "x = y?"=w299:bool)  [unwired: 8 in, 1 out]
                "ToolStringOut_P1" <- w297
                n130 = String Length(string=w297) -> (length=w295:i32)
                n131 = Not(x=w299) -> (.not. x?=w298:bool)
                n132 = Not Equal To 0?(x=w295) -> (x != 0?=w294:bool)
                n133 = Not(x=w294) -> (.not. x?=w296:bool)
                n134 = call "Retry Num.vi"("String"=w317) -> ("Numeric"=w324:i32, "retry次數"=w321:string[])  [unwired: 9 in]
                n135 = Or(x=w298, y=w296) -> ()  [unwired: 1 out]
                n136 = local write "retry次數"(w321) -> ()
                n137 = call "ToolProgramTest.vi"("error in (no error)"=w280, "VISA resource name"=w282) -> ("error out"=w279:errorcluster, "Array"=w293:string[])  [unwired: 4 in, 4 out]
                "P1 Receive" <- w293
                n138 = local write "Retry"(w324) -> ()
                n139 = Index Array(array=w293, index=0) -> (element=w291:string)
                n140 = Merge Errors(w279, w280) -> (w278:errorcluster)
                n141 = call "befor_ChkSum.vi"("ToolString Input"=w291) -> ("Array"=w290:string[])  [unwired: 9 in, 1 out]
                n142 = Unbundle By Name(w278) -> ("status"=w275:bool)
                n143 = call "Check Sum Test_01.vi"("Array"=w290) -> ("ToolStringOut_01"=w286:string, "x = y?"=w287:bool)  [unwired: 8 in, 1 out]
                "ToolStringOut_P1_2" <- w286
                n144 = String Length(string=w286) -> (length=w288:i32)
                n145 = Not(x=w287) -> (.not. x?=w285:bool)
                n146 = call "Get ProgReturn Info.vi"("String"=w286) -> ("Chk OK or Fail"=w281:bool)  [unwired: 8 in, 2 out]
                n147 = Not Equal To 0?(x=w288) -> (x != 0?=w289:bool)
                n148 = Select(t="OK" ("DataIn"), s=w281, f="NG" ("DataIn")) -> (s? t:f=w308:string)
                n149 = global read "Main Glb.vi" "Input Registers0-99"() -> (w302:u16[])
                n150 = Not(x=w289) -> (.not. x?=w284:bool)
                n151 = Compound Arithmetic op=OR(invert w281, w285, w284) -> (w277:bool)
                n152 = Compound Arithmetic op=OR(w277, w275) -> (w276:bool)
                n153 = Not(x=w276) -> (.not. x?=w272:bool)
                n154 = call "Red PLC InReg.vi"("length"=10, "index"=30, "Input Registers Arr"=w302) -> ("Rad In Reg"=w269:string)  [unwired: 7 in, 1 out]
                n155 = Increment(x=w316) -> (x+1=w325:i32)
                n156 = call "Cub Meaasure FGV.vi"("Action"=Table_Save."Write" ("Enum"), "Save Index"=MeasureDisplayTab."Programe(Tool Programe)", "DataIn"=w308, "SN"=w269) -> ()  [unwired: 8 in, 8 out]
                n157 = Select(t=w325, s=w276, f=w316) -> (s? t:f=w322:i32)
                n158 = case shown="False" w272 {
                  frame False {
                    n159 = call "Auto Inspection_Status.vi"("Action"=enum16{"Initial", "Write", "Read"}."Write", "DataIn"="PROGRAM1 RETRY", "Station"=Auto_Inspection_Station_Name2."S3Measure", "Data"=Auto_Inspection_Data_Name."ItemSN(TimeCode)") -> ()  [unwired: 9 in, 3 out]
                  }
                  frame True {
                  }
                }
                n160 = Increment(x=w318) -> (x+1=w326:i32)
                n161 = Select(t=w326, s=w272, f=w318) -> (s? t:f=w314:i32)
                n162 = Greater Or Equal?(x=w322, y=w324) -> (x >= y?=w323:bool)
                n163 = global write "Main Glb.vi" "S3 Barcode ID"(w269) -> ()
                n164 = case shown="True" w323 {
                  tunnel: [errorcluster {"status"=FALSE, "code"=0, "source"=""} ("error constant") errorcluster {"status"=TRUE, "code"=18302, "source"=""} ("error constant")] -> w274
                  tunnel: w322 -> [w354 _]
                  tunnel: [w354 0] -> w315
                  frame False {
                  }
                  frame True {
                  }
                }
                n165 = call "Cub Meaasure FGV.vi"("Action"=Table_Save."REad" ("Enum"), "Save Index"=MeasureDisplayTab."Tray Barcode", "SN"=w269) -> ("Read Index Data"=w268:string)  [unwired: 9 in, 7 out]
                n166 = global write "Main Glb.vi" "S3 Tary ID"(w268) -> ()
                n167 = case shown="Error .." w274 {
                  frame No Error {
                    w341 = T9[] [enum."S3 燒入程式 此站執行_34", enum."S3 燒入程式 OK_35"] items=["S2站PC動作中_20", "電流量測完成產品OK_21", "電流量測完成產品NG_22", "S2站Format 執行_23", "S2 Format OK_24", "S2 Format NG_25", "S2站燒入執行_26", "S2站燒入OK_27", "S2站燒入NG_28", "S2站動作完成_29", "S3 PC動作中_30", "S3 Format 此站執行_31", "S3 Format OK_32", "S3 Format NG_33", "S3 燒入程式 此站執行_34", "S3 燒入程式 OK_35", "S3 燒入程式 NG_36", "S3 備用_37", "S3 備用_38", "S3 動作完成_39", "S4 PC動作中_40", "S4 量測完成 產品正常_41", "S4 量測完成 產品NG_42", "S4 Format 此站執行_43", "S4 Format OK_44", "S4 Format NG_45", "S4 燒入 此站不執行_46", "S4 燒入程式 OK_47", "S4 燒入程式 NG_48", "S4 藍芽Scan OK_49", "S4 藍芽Scan NG_50", "S4 動作完成_51", "給PLC要量電流訊號", "給PLC要量電壓訊號"]
                    n168 = global read "Process Global.vi" "S3Tool Action"() -> (w340:bool[])
                    n169 = call "Auto Inspection_Status.vi"("Action"=enum16{"Initial", "Write", "Read"}."Write", "DataIn"="PROGRAM1成功", "Station"=Auto_Inspection_Station_Name2."S3Measure", "Data"=Auto_Inspection_Data_Name."ItemSN(TimeCode)") -> ()  [unwired: 9 in, 3 out]
                    n170 = call "Set OutputPLC.vi"("Address In"=20, "Array 2"=w341, "Sat Coils"=bool[] [TRUE]) -> ()  [unwired: 7 in, 1 out]
                    n171 = Replace Array Subset(array=w340, new element=TRUE ("new element/subarray"), index=3) -> (w333:bool[])
                    n172 = global write "Process Global.vi" "S3Tool Action"(w333) -> ()
                  }
                  frame Error {
                    w353 = T9[] [enum."S3 燒入程式 此站執行_34", enum."S3 燒入程式 NG_36"] items=["S2站PC動作中_20", "電流量測完成產品OK_21", "電流量測完成產品NG_22", "S2站Format 執行_23", "S2 Format OK_24", "S2 Format NG_25", "S2站燒入執行_26", "S2站燒入OK_27", "S2站燒入NG_28", "S2站動作完成_29", "S3 PC動作中_30", "S3 Format 此站執行_31", "S3 Format OK_32", "S3 Format NG_33", "S3 燒入程式 此站執行_34", "S3 燒入程式 OK_35", "S3 燒入程式 NG_36", "S3 備用_37", "S3 備用_38", "S3 動作完成_39", "S4 PC動作中_40", "S4 量測完成 產品正常_41", "S4 量測完成 產品NG_42", "S4 Format 此站執行_43", "S4 Format OK_44", "S4 Format NG_45", "S4 燒入 此站不執行_46", "S4 燒入程式 OK_47", "S4 燒入程式 NG_48", "S4 藍芽Scan OK_49", "S4 藍芽Scan NG_50", "S4 動作完成_51", "給PLC要量電流訊號", "給PLC要量電壓訊號"]
                    n173 = global read "Process Global.vi" "S3Tool Action"() -> (w351:bool[])
                    n174 = call "Auto Inspection_Status.vi"("Action"=enum16{"Initial", "Write", "Read"}."Write", "DataIn"="PROGRAM1失敗", "Station"=Auto_Inspection_Station_Name2."S3Measure", "Data"=Auto_Inspection_Data_Name."ItemSN(TimeCode)") -> ()  [unwired: 9 in, 3 out]
                    n175 = call "Set OutputPLC.vi"("Address In"=20, "Array 2"=w353, "Sat Coils"=bool[] [TRUE]) -> ()  [unwired: 7 in, 1 out]
                    n176 = Replace Array Subset(array=w351, new element=FALSE ("new element/subarray"), index=3) -> (w344:bool[])
                    n177 = global write "Process Global.vi" "S3Tool Action"(w344) -> ()
                  }
                }
              }
              frame "P2" {
                # "經過燒錄後第二次Tool回傳"
                # "下Cmd後第一次Tool回傳"
                # "收尋S2站條碼"
                # "SEND RECEIVE Recore"
                n178 = Index Array(array=w375, index=StationCmdSelect."Command") -> (element=w365:string)
                n179 = call "Tool RS232 test for S3.vi"("error in (no error)"=w364, "Cmd In"=w365, "VISA resource name"=w376) -> ("error out"=w413:errorcluster, "receive string"=→"Program receive 2":string)  [unwired: 7 in]
                n180 = call "befor_ChkSum.vi"("ToolString Input"=w365) -> ("Array"=w396:string[])  [unwired: 9 in, 1 out]
                n181 = local write "CurrentCmd"(w365) -> ()
                n182 = call "Check Sum Test_01.vi"("Array"=w396) -> ("ToolStringOut_01"=w399:string, "x = y?"=w397:bool)  [unwired: 8 in, 1 out]
                "ToolStringOut_P1 2" <- w399
                n183 = call "Auto Inspection_Status.vi"("Action"=enum16{"Initial", "Write", "Read"}."Write", "DataIn"="PROGRAM2", "Station"=Auto_Inspection_Station_Name2."S3Measure", "Data"=Auto_Inspection_Data_Name."CurrentAction", "error in"=w364) -> ()  [unwired: 8 in, 3 out]
                n184 = String Length(string=w399) -> (length=w401:i32)
                n185 = Not(x=w397) -> (.not. x?=w398:bool)
                n186 = Not Equal To 0?(x=w401) -> (x != 0?=w402:bool)
                n187 = Not(x=w402) -> (.not. x?=w400:bool)
                n188 = call "Retry Num.vi"("String"=w374) -> ("Numeric"=w366:i32, "retry次數"=w367:string[])  [unwired: 9 in]
                n189 = Or(x=w398, y=w400) -> ()  [unwired: 1 out]
                n190 = local write "retry次數"(w367) -> ()
                n191 = local write "Retry"(w366) -> ()
                n192 = call "ToolProgramTest.vi"("error in (no error)"=w413, "VISA resource name"=w376) -> ("error out"=w414:errorcluster, "Array"=w403:string[])  [unwired: 4 in, 4 out]
                "P1 Receive 2" <- w403
                n193 = Index Array(array=w403, index=0) -> (element=w404:string)
                n194 = Merge Errors(w414, w413) -> (w415:errorcluster)
                n195 = call "befor_ChkSum.vi"("ToolString Input"=w404) -> ("Array"=w405:string[])  [unwired: 9 in, 1 out]
                n196 = Unbundle By Name(w415) -> ("status"=w418:bool)
                n197 = call "Check Sum Test_01.vi"("Array"=w405) -> ("ToolStringOut_01"=w409:string, "x = y?"=w408:bool)  [unwired: 8 in, 1 out]
                "ToolStringOut_P1_2 2" <- w409
                n198 = String Length(string=w409) -> (length=w407:i32)
                n199 = Not(x=w408) -> (.not. x?=w410:bool)
                n200 = call "Get ProgReturn Info.vi"("String"=w409) -> ("Chk OK or Fail"=w412:bool)  [unwired: 8 in, 2 out]
                n201 = Not Equal To 0?(x=w407) -> (x != 0?=w406:bool)
                n202 = Select(t="OK" ("DataIn"), s=w412, f="NG" ("DataIn")) -> (s? t:f=w394:string)
                n203 = global read "Main Glb.vi" "Input Registers0-99"() -> (w395:u16[])
                n204 = Not(x=w406) -> (.not. x?=w411:bool)
                n205 = Compound Arithmetic op=OR(invert w412, w410, w411) -> (w416:bool)
                n206 = Compound Arithmetic op=OR(w416, w418) -> (w417:bool)
                n207 = Not(x=w417) -> (.not. x?=w363:bool)
                n208 = call "Red PLC InReg.vi"("length"=10, "index"=30, "Input Registers Arr"=w395) -> ("Rad In Reg"=w360:string)  [unwired: 7 in, 1 out]
                n209 = Increment(x=w373) -> (x+1=w391:i32)
                n210 = case shown="False" w363 {
                  frame False {
                    n211 = call "Auto Inspection_Status.vi"("Action"=enum16{"Initial", "Write", "Read"}."Write", "DataIn"="PROGRAM2 RETRY", "Station"=Auto_Inspection_Station_Name2."S3Measure", "Data"=Auto_Inspection_Data_Name."ItemSN(TimeCode)") -> ()  [unwired: 9 in, 3 out]
                  }
                  frame True {
                  }
                }
                n212 = call "Cub Meaasure FGV.vi"("Action"=Table_Save."Write" ("Enum"), "Save Index"=MeasureDisplayTab."Programe(Tool Programe)", "DataIn"=w394, "SN"=w360) -> ("error out"=w359:errorcluster)  [unwired: 8 in, 7 out]
                n213 = Select(t=w391, s=w417, f=w373) -> (s? t:f=w393:i32)
                n214 = Increment(x=w371) -> (x+1=w390:i32)
                n215 = Select(t=w390, s=w363, f=w371) -> (s? t:f=w372:i32)
                n216 = Greater Or Equal?(x=w393, y=w366) -> (x >= y?=w392:bool)
                n217 = global write "Main Glb.vi" "S3 Barcode ID"(w360) -> ()
                n218 = call "Cub Meaasure FGV.vi"("Action"=Table_Save."REad" ("Enum"), "Save Index"=MeasureDisplayTab."Tray Barcode", "SN"=w360, "error in (no error)"=w359) -> ("Read Index Data"=w358:string)  [unwired: 8 in, 7 out]
                n219 = case shown="True" w392 {
                  tunnel: [errorcluster {"status"=FALSE, "code"=0, "source"=""} ("error constant") errorcluster {"status"=TRUE, "code"=18302, "source"=""} ("error constant")] -> w368
                  tunnel: w393 -> [w446 _]
                  tunnel: [w446 0] -> w369
                  frame False {
                  }
                  frame True {
                  }
                }
                n220 = global write "Main Glb.vi" "S3 Tary ID"(w358) -> ()
                n221 = case shown="Error .." w368 {
                  tunnel: w363 -> [w423 _]
                  frame No Error {
                    n222 = case shown="True" w423 {
                      frame False {
                      }
                      frame True {
                        w433 = T9[] [enum."S3 燒入程式 此站執行_34", enum."S3 燒入程式 OK_35"] items=["S2站PC動作中_20", "電流量測完成產品OK_21", "電流量測完成產品NG_22", "S2站Format 執行_23", "S2 Format OK_24", "S2 Format NG_25", "S2站燒入執行_26", "S2站燒入OK_27", "S2站燒入NG_28", "S2站動作完成_29", "S3 PC動作中_30", "S3 Format 此站執行_31", "S3 Format OK_32", "S3 Format NG_33", "S3 燒入程式 此站執行_34", "S3 燒入程式 OK_35", "S3 燒入程式 NG_36", "S3 備用_37", "S3 備用_38", "S3 動作完成_39", "S4 PC動作中_40", "S4 量測完成 產品正常_41", "S4 量測完成 產品NG_42", "S4 Format 此站執行_43", "S4 Format OK_44", "S4 Format NG_45", "S4 燒入 此站不執行_46", "S4 燒入程式 OK_47", "S4 燒入程式 NG_48", "S4 藍芽Scan OK_49", "S4 藍芽Scan NG_50", "S4 動作完成_51", "給PLC要量電流訊號", "給PLC要量電壓訊號"]
                        n223 = global read "Process Global.vi" "S3Tool Action"() -> (w432:bool[])
                        n224 = call "Auto Inspection_Status.vi"("Action"=enum16{"Initial", "Write", "Read"}."Write", "DataIn"="PROGRAM2 成功", "Station"=Auto_Inspection_Station_Name2."S3Measure", "Data"=Auto_Inspection_Data_Name."ItemSN(TimeCode)") -> ()  [unwired: 9 in, 3 out]
                        n225 = call "Set OutputPLC.vi"("Address In"=20, "Array 2"=w433, "Sat Coils"=bool[] [TRUE]) -> ()  [unwired: 7 in, 1 out]
                        n226 = Replace Array Subset(array=w432, new element=TRUE ("new element/subarray"), index=3) -> (w425:bool[])
                        n227 = global write "Process Global.vi" "S3Tool Action"(w425) -> ()
                      }
                    }
                  }
                  frame Error {
                    w445 = T9[] [enum."S3 燒入程式 此站執行_34", enum."S3 燒入程式 NG_36"] items=["S2站PC動作中_20", "電流量測完成產品OK_21", "電流量測完成產品NG_22", "S2站Format 執行_23", "S2 Format OK_24", "S2 Format NG_25", "S2站燒入執行_26", "S2站燒入OK_27", "S2站燒入NG_28", "S2站動作完成_29", "S3 PC動作中_30", "S3 Format 此站執行_31", "S3 Format OK_32", "S3 Format NG_33", "S3 燒入程式 此站執行_34", "S3 燒入程式 OK_35", "S3 燒入程式 NG_36", "S3 備用_37", "S3 備用_38", "S3 動作完成_39", "S4 PC動作中_40", "S4 量測完成 產品正常_41", "S4 量測完成 產品NG_42", "S4 Format 此站執行_43", "S4 Format OK_44", "S4 Format NG_45", "S4 燒入 此站不執行_46", "S4 燒入程式 OK_47", "S4 燒入程式 NG_48", "S4 藍芽Scan OK_49", "S4 藍芽Scan NG_50", "S4 動作完成_51", "給PLC要量電流訊號", "給PLC要量電壓訊號"]
                    n228 = global read "Process Global.vi" "S3Tool Action"() -> (w443:bool[])
                    n229 = call "Auto Inspection_Status.vi"("Action"=enum16{"Initial", "Write", "Read"}."Write", "DataIn"="PROGRAM2 失敗", "Station"=Auto_Inspection_Station_Name2."S3Measure", "Data"=Auto_Inspection_Data_Name."ItemSN(TimeCode)") -> ()  [unwired: 9 in, 3 out]
                    n230 = Replace Array Subset(array=w443, new element=FALSE ("new element/subarray"), index=3) -> (w436:bool[])
                    n231 = call "Set OutputPLC.vi"("Address In"=20, "Array 2"=w445, "Sat Coils"=bool[] [TRUE]) -> ()  [unwired: 7 in, 1 out]
                    n232 = global write "Process Global.vi" "S3Tool Action"(w436) -> ()
                  }
                }
              }
              frame "S1" {
                # "收尋S3站條碼"
                n233 = call "Retry Num.vi"("String"=w498) -> ("Numeric"=w488:i32, "retry次數"=w485:string[])  [unwired: 9 in]
                n234 = Index Array(array=w497, index=StationCmdSelect."Command") -> (element=w483:string)
                n235 = call "Auto Inspection_Status.vi"("Action"=enum16{"Initial", "Write", "Read"}."Write", "DataIn"="SCAN1", "Station"=Auto_Inspection_Station_Name2."S3Measure", "Data"=Auto_Inspection_Data_Name."CurrentAction") -> ()  [unwired: 9 in, 3 out]
                n236 = call "Tool RS232 test for S3.vi"("error in (no error)"=w452, "Cmd In"=w483, "VISA resource name"=w465) -> ("error out"=w491:errorcluster, "receive string"=→"S1 receive":string)  [unwired: 7 in]
                n237 = local write "CurrentCmd"(w483) -> ()
                n238 = local write "retry次數"(w485) -> ()
                n239 = local write "Retry"(w488) -> ()
                n240 = call "ToolScanTest.vi"("error in (no error)"=w452, "VISA resource name"=refnum<visa-resource-name> "COM10") -> ("error out"=w462:errorcluster, "read string 6"=w458:string, "Array"=w459:string[])  [unwired: 4 in, 3 out]
                "Blue Scan receive" <- w458
                "Array" <- w459
                n241 = Unbundle By Name(w491) -> ("status"=w482:bool)
                n242 = String Length(string=w458) -> (length=w457:i32)
                n243 = call <vilib>:"Clear Errors.vi"("error in (no error)"=w462) -> ()  [unwired: 5 in, 2 out]
                n244 = Not Equal?(x=w457, y=0) -> (x != y?=w455:bool)
                n245 = call "Check Sum Test_01.vi"("Array"=w459) -> ("ToolStringOut_01"=→"S1 ToolStringOut":string, "ChkSum"=→"S1 ChkSum":string, "x = y?"=w461:bool)  [unwired: 8 in]
                n246 = Not(x=w455) -> (.not. x?=w454:bool)
                n247 = Not(x=w461) -> (.not. x?=w453:bool)
                n248 = Or(x=w453, y=w454) -> (x .or. y?=w451:bool)
                n249 = Or(x=w451, y=w482) -> (x .or. y?=w481:bool)
                n250 = Not(x=w481) -> (.not. x?=w450:bool)
                n251 = Increment(x=w495) -> (x+1=w489:i32)
                n252 = Select(t=w489, s=w481, f=w495) -> (s? t:f=w486:i32)
                n253 = Increment(x=w496) -> (x+1=w490:i32)
                n254 = Greater Or Equal?(x=w486, y=w488) -> (x >= y?=w487:bool)
                n255 = Select(t=w490, s=w450, f=w496) -> (s? t:f=w500:i32)
                n256 = disable-structure shown="Disabled" {
                  disable-tunnel: [w502 _] -> w480
                  disable-tunnel: _ -> [w501 _]
                  frame Disabled {
                    n257 = case shown="True" w501 {
                      tunnel: [w503 w507] -> w502
                      frame False {
                        w505 = T9[] [enum."S4 量測完成 產品NG_42"] items=["S2站PC動作中_20", "電流量測完成產品OK_21", "電流量測完成產品NG_22", "S2站Format 執行_23", "S2 Format OK_24", "S2 Format NG_25", "S2站燒入執行_26", "S2站燒入OK_27", "S2站燒入NG_28", "S2站動作完成_29", "S3 PC動作中_30", "S3 Format 此站執行_31", "S3 Format OK_32", "S3 Format NG_33", "S3 燒入程式 此站執行_34", "S3 燒入程式 OK_35", "S3 燒入程式 NG_36", "S3 備用_37", "S3 備用_38", "S3 動作完成_39", "S4 PC動作中_40", "S4 量測完成 產品正常_41", "S4 量測完成 產品NG_42", "S4 Format 此站執行_43", "S4 Format OK_44", "S4 Format NG_45", "S4 燒入 此站不執行_46", "S4 燒入程式 OK_47", "S4 燒入程式 NG_48", "S4 藍芽Scan OK_49", "S4 藍芽Scan NG_50", "S4 動作完成_51", "給PLC要量電流訊號", "給PLC要量電壓訊號"]
                        n258 = call "Set OutputPLC.vi"("Array"=w505, "Address In"=20) -> ("Error Out"=w503:errorcluster[])  [unwired: 9 in]
                      }
                      frame True {
                        w506 = T9[] [enum."S4 量測完成 產品正常_41"] items=["S2站PC動作中_20", "電流量測完成產品OK_21", "電流量測完成產品NG_22", "S2站Format 執行_23", "S2 Format OK_24", "S2 Format NG_25", "S2站燒入執行_26", "S2站燒入OK_27", "S2站燒入NG_28", "S2站動作完成_29", "S3 PC動作中_30", "S3 Format 此站執行_31", "S3 Format OK_32", "S3 Format NG_33", "S3 燒入程式 此站執行_34", "S3 燒入程式 OK_35", "S3 燒入程式 NG_36", "S3 備用_37", "S3 備用_38", "S3 動作完成_39", "S4 PC動作中_40", "S4 量測完成 產品正常_41", "S4 量測完成 產品NG_42", "S4 Format 此站執行_43", "S4 Format OK_44", "S4 Format NG_45", "S4 燒入 此站不執行_46", "S4 燒入程式 OK_47", "S4 燒入程式 NG_48", "S4 藍芽Scan OK_49", "S4 藍芽Scan NG_50", "S4 動作完成_51", "給PLC要量電流訊號", "給PLC要量電壓訊號"]
                        n259 = call "Set OutputPLC.vi"("Array"=w506, "Address In"=20) -> ("Error Out"=w507:errorcluster[])  [unwired: 9 in]
                      }
                    }
                  }
                  frame Enabled {
                  }
                }
                n260 = global read "Main Glb.vi" "Input Registers0-99"() -> (w467:u16[])
                n261 = Select(t="OK" ("DataIn"), s=w450, f="NG" ("DataIn")) -> (s? t:f=w474:string)
                n262 = case shown="True" w487 {
                  tunnel: [errorcluster {"status"=FALSE, "code"=0, "source"=""} ("error constant") errorcluster {"status"=TRUE, "code"=18303, "source"=""} ("error constant")] -> w479
                  tunnel: w486 -> [w509 _]
                  tunnel: [w509 0] -> w499
                  frame False {
                  }
                  frame True {
                  }
                }
                n263 = call "Red PLC InReg.vi"("length"=10, "index"=30, "Input Registers Arr"=w467) -> ("Rad In Reg"=w468:string)  [unwired: 7 in, 1 out]
                n264 = call "Cub Meaasure FGV.vi"("Action"=Table_Save."Write" ("Enum"), "Save Index"=MeasureDisplayTab."FSKscanl_315(FSK scan)", "DataIn"=w474, "SN"=w468) -> ()  [unwired: 8 in, 8 out]
                n265 = Merge Errors(w480, w479) -> (w493:errorcluster)
              }
              frame "S2" {
                # "藍芽接收"
                # "收尋S3站條碼"
                n266 = call "Retry Num.vi"("String"=w552) -> ("Numeric"=w543:i32, "retry次數"=w540:string[])  [unwired: 9 in]
                n267 = Index Array(array=w553, index=StationCmdSelect."Command") -> (element=w539:string)
                n268 = call "ToolScanTest.vi"("error in (no error)"=w554, "VISA resource name"=refnum<visa-resource-name> "COM10") -> ("error out"=w538:errorcluster, "read string 3"=w536:string)  [unwired: 4 in, 4 out]
                "Blue Scan2 receive" <- w536
                n269 = local write "retry次數"(w540) -> ()
                n270 = call "Tool RS232 test for S3.vi"("error in (no error)"=w554, "Cmd In"=w539, "VISA resource name"=w513) -> ("error out"=w546:errorcluster, "receive string"=→"S2 receive":string)  [unwired: 7 in]
                n271 = local write "CurrentCmd"(w539) -> ()
                n272 = call <vilib>:"Clear Errors.vi"("error in (no error)"=w538) -> ()  [unwired: 5 in, 2 out]
                n273 = local write "Retry"(w543) -> ()
                n274 = Unbundle By Name(w546) -> ("status"=w533:bool)
                n275 = String Length(string=w536) -> (length=w537:i32)
                n276 = Not Equal To 0?(x=w537) -> (x != 0?=w535:bool)
                n277 = Not(x=w535) -> (.not. x?=w534:bool)
                n278 = Or(x=w534, y=w533) -> (x .or. y?=w532:bool)
                n279 = Not(x=w532) -> (.not. x?=w515:bool)
                n280 = Increment(x=w551) -> (x+1=w544:i32)
                n281 = call "Auto Inspection_Status.vi"("Action"=enum16{"Initial", "Write", "Read"}."Write", "DataIn"="SCAN2", "Station"=Auto_Inspection_Station_Name2."S3Measure", "Data"=Auto_Inspection_Data_Name."CurrentAction") -> ()  [unwired: 9 in, 3 out]
                n282 = Select(t=w544, s=w532, f=w551) -> (s? t:f=w541:i32)
                n283 = Increment(x=w555) -> (x+1=w545:i32)
                n284 = Greater Or Equal?(x=w541, y=w543) -> (x >= y?=w542:bool)
                n285 = Select(t=w545, s=w515, f=w555) -> (s? t:f=w550:i32)
                n286 = disable-structure shown="Disabled" {
                  disable-tunnel: [w558 _] -> w529
                  disable-tunnel: w515 -> [w557 _]
                  frame Disabled {
                    n287 = case shown="True" w557 {
                      tunnel: [w559 w563] -> w558
                      frame False {
                        w561 = T9[] [enum."S4 量測完成 產品NG_42"] items=["S2站PC動作中_20", "電流量測完成產品OK_21", "電流量測完成產品NG_22", "S2站Format 執行_23", "S2 Format OK_24", "S2 Format NG_25", "S2站燒入執行_26", "S2站燒入OK_27", "S2站燒入NG_28", "S2站動作完成_29", "S3 PC動作中_30", "S3 Format 此站執行_31", "S3 Format OK_32", "S3 Format NG_33", "S3 燒入程式 此站執行_34", "S3 燒入程式 OK_35", "S3 燒入程式 NG_36", "S3 備用_37", "S3 備用_38", "S3 動作完成_39", "S4 PC動作中_40", "S4 量測完成 產品正常_41", "S4 量測完成 產品NG_42", "S4 Format 此站執行_43", "S4 Format OK_44", "S4 Format NG_45", "S4 燒入 此站不執行_46", "S4 燒入程式 OK_47", "S4 燒入程式 NG_48", "S4 藍芽Scan OK_49", "S4 藍芽Scan NG_50", "S4 動作完成_51", "給PLC要量電流訊號", "給PLC要量電壓訊號"]
                        n288 = call "Set OutputPLC.vi"("Array"=w561, "Address In"=20) -> ("Error Out"=w559:errorcluster[])  [unwired: 9 in]
                      }
                      frame True {
                        w562 = T9[] [enum."S4 量測完成 產品正常_41"] items=["S2站PC動作中_20", "電流量測完成產品OK_21", "電流量測完成產品NG_22", "S2站Format 執行_23", "S2 Format OK_24", "S2 Format NG_25", "S2站燒入執行_26", "S2站燒入OK_27", "S2站燒入NG_28", "S2站動作完成_29", "S3 PC動作中_30", "S3 Format 此站執行_31", "S3 Format OK_32", "S3 Format NG_33", "S3 燒入程式 此站執行_34", "S3 燒入程式 OK_35", "S3 燒入程式 NG_36", "S3 備用_37", "S3 備用_38", "S3 動作完成_39", "S4 PC動作中_40", "S4 量測完成 產品正常_41", "S4 量測完成 產品NG_42", "S4 Format 此站執行_43", "S4 Format OK_44", "S4 Format NG_45", "S4 燒入 此站不執行_46", "S4 燒入程式 OK_47", "S4 燒入程式 NG_48", "S4 藍芽Scan OK_49", "S4 藍芽Scan NG_50", "S4 動作完成_51", "給PLC要量電流訊號", "給PLC要量電壓訊號"]
                        n289 = call "Set OutputPLC.vi"("Array"=w562, "Address In"=20) -> ("Error Out"=w563:errorcluster[])  [unwired: 9 in]
                      }
                    }
                  }
                  frame Enabled {
                  }
                }
                n290 = case shown="True" w542 {
                  tunnel: [errorcluster {"status"=FALSE, "code"=0, "source"=""} ("error constant") errorcluster {"status"=TRUE, "code"=18304, "source"=""} ("error constant")] -> w528
                  tunnel: w541 -> [w565 _]
                  tunnel: [w565 0] -> w549
                  frame False {
                  }
                  frame True {
                  }
                }
                n291 = Merge Errors(w529, w528) -> (w548:errorcluster)
                n292 = Select(t="OK" ("DataIn"), s=w515, f="NG" ("DataIn")) -> (s? t:f=w523:string)
                n293 = global read "Main Glb.vi" "Input Registers0-99"() -> (w516:u16[])
                n294 = call "Red PLC InReg.vi"("length"=10, "index"=30, "Input Registers Arr"=w516) -> ("Rad In Reg"=w517:string)  [unwired: 7 in, 1 out]
                n295 = call "Cub Meaasure FGV.vi"("Action"=Table_Save."Write" ("Enum"), "Save Index"=MeasureDisplayTab."ASKscan_433(ASK scan)", "DataIn"=w523, "SN"=w517) -> ()  [unwired: 8 in, 8 out]
              }
              frame "D" {
                n296 = Index Array(array=w580) -> (element=w579:i32)  [unwired: 1 in]
                n297 = Multiply(x=1000, y=w579) -> (x*y=w578:i32)
                n298 = Wait (ms)(milliseconds to wait=w578) -> ()  [unwired: 1 out]
                n299 = Increment(x=w575) -> (x+1=w574:i32)
                n300 = call "Auto Inspection_Status.vi"("Action"=enum16{"Initial", "Write", "Read"}."Write", "DataIn"="Delay", "Station"=Auto_Inspection_Station_Name2."S3Measure", "Data"=Auto_Inspection_Data_Name."CurrentAction") -> ()  [unwired: 9 in, 3 out]
              }
              frame "T1" {
                w585 = T9[] [enum."給PLC要量電壓訊號"] items=["S2站PC動作中_20", "電流量測完成產品OK_21", "電流量測完成產品NG_22", "S2站Format 執行_23", "S2 Format OK_24", "S2 Format NG_25", "S2站燒入執行_26", "S2站燒入OK_27", "S2站燒入NG_28", "S2站動作完成_29", "S3 PC動作中_30", "S3 Format 此站執行_31", "S3 Format OK_32", "S3 Format NG_33", "S3 燒入程式 此站執行_34", "S3 燒入程式 OK_35", "S3 燒入程式 NG_36", "S3 備用_37", "S3 備用_38", "S3 動作完成_39", "S4 PC動作中_40", "S4 量測完成 產品正常_41", "S4 量測完成 產品NG_42", "S4 Format 此站執行_43", "S4 Format OK_44", "S4 Format NG_45", "S4 燒入 此站不執行_46", "S4 燒入程式 OK_47", "S4 燒入程式 NG_48", "S4 藍芽Scan OK_49", "S4 藍芽Scan NG_50", "S4 動作完成_51", "給PLC要量電流訊號", "給PLC要量電壓訊號"]
                n301 = flat-sequence {
                  tunnel: [w594] -> w586
                  tunnel: w583 -> [_]
                  frame #0 {
                    n302 = global read "Main Glb.vi" "Discrete Inputs"() -> (w596:bool[])
                    n303 = Index Array(array=w596, index=S2_Station_Input."21_PLC下達可測電流訊號" ("Enum")) -> (element=w594:bool)
                  }
                }
                n304 = call "Set OutputPLC.vi"("Address In"=20, "Array 2"=w585, "Sat Coils"=bool[] [TRUE]) -> ("Error Out"=w583:errorcluster[])  [unwired: 7 in]
                n305 = case shown="True" w586 {
                  tunnel: w592 -> [_ w635]
                  tunnel: w591 -> [_ w634]
                  tunnel: [0 ("Err Count") w632] -> w590
                  tunnel: w589 -> [w604 w631]
                  tunnel: [w604 w629] -> w588
                  tunnel: [errorcluster {"status"=FALSE, "code"=0, "source"=""} ("error IO") w605] -> w587
                  frame False {
                    n306 = call "Auto Inspection_Status.vi"("Action"=enum16{"Initial", "Write", "Read"}."Write", "DataIn"="等待PLC可量電流訊號", "Station"=Auto_Inspection_Station_Name2."S3Measure", "Data"=Auto_Inspection_Data_Name."CurrentAction") -> ()  [unwired: 9 in, 3 out]
                    n307 = Wait (ms)(milliseconds to wait=250) -> ()  [unwired: 1 out]
                  }
                  frame True {
                    w639 = u16 3 items=["SYSTem:VERSion?", "SYSTem:ERRor?", "*IDN?", "MEAS:CURR:DC?", "MEAS:VOLT?", "SYSTem:ERRor?"] ("Ringfor34450A")
                    w638 = u16 5 items=["SYSTem:VERSion?", "SYSTem:ERRor?", "*IDN?", "MEAS:CURR:DC?", "MEAS:VOLT?", "MEAS:VOLT:DC?"] ("RingforIT8511")
                    w636 = u16 1 items=["IT8511", "34450A", "WRBuff"] ("ChangeStatus")
                    # "收尋S3站條碼"
                    # "T1 34450A/"
                    # "量電流"
                    n308 = call "Retry Num.vi"("String"=w634) -> ("Numeric"=w641:i32, "retry次數"=w640:string[])  [unwired: 9 in]
                    n309 = call "Auto Inspection_Status.vi"("Action"=enum16{"Initial", "Write", "Read"}."Write", "DataIn"="儀器測量中", "Station"=Auto_Inspection_Station_Name2."S3Measure", "Data"=Auto_Inspection_Data_Name."CurrentAction") -> ()  [unwired: 9 in, 3 out]
                    n310 = local write "retry次數"(w640) -> ()
                    n311 = local write "Retry"(w641) -> ()
                    n312 = call "MTool34450A.vi"("Ringfor34450A"=w639, "RingforIT8511"=w638, "VISA resource name"=refnum<visa-resource-name> "USB0::0x2A8D::0xB318::MY59430005::INSTR", "ChangeStatus"=w636) -> ("error out"=w627:errorcluster, 1:"μA"=w610:string, 2:"μA"=→"T1 μA":dbl, "read buffer"=w624:string)  [unwired: 4 in]
                    "T1 buffer" <- w624
                    n313 = Unbundle By Name(w627) -> ("status"=w630:bool)
                    n314 = Increment(x=w635) -> (x+1=w642:i32)
                    n315 = Select(t=w642, s=w630, f=w635) -> (s? t:f=w633:i32)
                    n316 = Greater Or Equal?(x=w633, y=w641) -> (x >= y?=w628:bool)
                    n317 = call "AL量測值轉換.vi"("位數"=4, "input string"=w624, "PLC address"=20) -> ("error out"=w618:errorcluster)  [unwired: 7 in, 1 out]
                    n318 = Not(x=w630) -> (.not. x?=w609:bool)
                    n319 = case shown="True" w628 {
                      tunnel: [errorcluster {"status"=FALSE, "code"=0, "source"=""} ("error constant") errorcluster {"status"=TRUE, "code"=18305, "source"=""} ("error constant")] -> w623
                      tunnel: w633 -> [w661 _]
                      tunnel: [w661 0] -> w632
                      tunnel: w627 -> [_ _]
                      frame False {
                      }
                      frame True {
                      }
                    }
                    n320 = Increment(x=w631) -> (x+1=w643:i32)
                    n321 = Select(t=w643, s=w609, f=w631) -> (s? t:f=w629:i32)
                    n322 = disable-structure shown="Disabled" {
                      disable-tunnel: w609 -> [w654 _]
                      disable-tunnel: [w653 _] -> w608
                      frame Disabled {
                        n323 = case shown="True" w654 {
                          tunnel: [w655 w658] -> w653
                          frame False {
                            w657 = T9[] [enum."電流量測完成產品NG_22"] items=["S2站PC動作中_20", "電流量測完成產品OK_21", "電流量測完成產品NG_22", "S2站Format 執行_23", "S2 Format OK_24", "S2 Format NG_25", "S2站燒入執行_26", "S2站燒入OK_27", "S2站燒入NG_28", "S2站動作完成_29", "S3 PC動作中_30", "S3 Format 此站執行_31", "S3 Format OK_32", "S3 Format NG_33", "S3 燒入程式 此站執行_34", "S3 燒入程式 OK_35", "S3 燒入程式 NG_36", "S3 備用_37", "S3 備用_38", "S3 動作完成_39", "S4 PC動作中_40", "S4 量測完成 產品正常_41", "S4 量測完成 產品NG_42", "S4 Format 此站執行_43", "S4 Format OK_44", "S4 Format NG_45", "S4 燒入 此站不執行_46", "S4 燒入程式 OK_47", "S4 燒入程式 NG_48", "S4 藍芽Scan OK_49", "S4 藍芽Scan NG_50", "S4 動作完成_51", "給PLC要量電流訊號", "給PLC要量電壓訊號"]
                            n324 = call "Set OutputPLC.vi"("Array"=w657, "Address In"=20) -> ("Error Out"=w655:errorcluster[])  [unwired: 9 in]
                          }
                          frame True {
                            w659 = T9[] [enum."電流量測完成產品OK_21"] items=["S2站PC動作中_20", "電流量測完成產品OK_21", "電流量測完成產品NG_22", "S2站Format 執行_23", "S2 Format OK_24", "S2 Format NG_25", "S2站燒入執行_26", "S2站燒入OK_27", "S2站燒入NG_28", "S2站動作完成_29", "S3 PC動作中_30", "S3 Format 此站執行_31", "S3 Format OK_32", "S3 Format NG_33", "S3 燒入程式 此站執行_34", "S3 燒入程式 OK_35", "S3 燒入程式 NG_36", "S3 備用_37", "S3 備用_38", "S3 動作完成_39", "S4 PC動作中_40", "S4 量測完成 產品正常_41", "S4 量測完成 產品NG_42", "S4 Format 此站執行_43", "S4 Format OK_44", "S4 Format NG_45", "S4 燒入 此站不執行_46", "S4 燒入程式 OK_47", "S4 燒入程式 NG_48", "S4 藍芽Scan OK_49", "S4 藍芽Scan NG_50", "S4 動作完成_51", "給PLC要量電流訊號", "給PLC要量電壓訊號"]
                            n325 = call "Set OutputPLC.vi"("Array"=w659, "Address In"=20) -> ("Error Out"=w658:errorcluster[])  [unwired: 9 in]
                          }
                        }
                      }
                      frame Enabled {
                      }
                    }
                    n326 = Select(t=w610, s=w609, f="NG" ("DataIn")) -> (s? t:f=w617:string)
                    n327 = global read "Main Glb.vi" "Input Registers0-99"() -> (w611:u16[])
                    n328 = Merge Errors(w618, w623) -> (w607:errorcluster)
                    n329 = call "Red PLC InReg.vi"("length"=10, "index"=30, "Input Registers Arr"=w611) -> ("Rad In Reg"=w612:string)  [unwired: 7 in, 1 out]
                    n330 = call "Cub Meaasure FGV.vi"("Action"=Table_Save."Write" ("Enum"), "Save Index"=MeasureDisplayTab."耗電流 uA(電流表)", "DataIn"=w617, "SN"=w612) -> ()  [unwired: 8 in, 8 out]
                    n331 = Merge Errors(w608, w607) -> (w605:errorcluster)
                    n332 = case shown="Error .." w605 {
                      frame No Error {
                        n333 = global read "Process Global.vi" "S3Tool Action"() -> (w647:bool[])
                        n334 = Replace Array Subset(array=w647, new element=TRUE ("new element/subarray"), index=5) -> (w648:bool[])
                        n335 = global write "Process Global.vi" "S3Tool Action"(w648) -> ()
                      }
                      frame Error {
                        n336 = global read "Process Global.vi" "S3Tool Action"() -> (w651:bool[])
                        n337 = Replace Array Subset(array=w651, new element=FALSE ("new element/subarray"), index=5) -> (w652:bool[])
                        n338 = global write "Process Global.vi" "S3Tool Action"(w652) -> ()
                      }
                    }
                  }
                }
              }
              frame "T2" {
                w668 = T9[] [enum."給PLC要量電壓訊號"] items=["S2站PC動作中_20", "電流量測完成產品OK_21", "電流量測完成產品NG_22", "S2站Format 執行_23", "S2 Format OK_24", "S2 Format NG_25", "S2站燒入執行_26", "S2站燒入OK_27", "S2站燒入NG_28", "S2站動作完成_29", "S3 PC動作中_30", "S3 Format 此站執行_31", "S3 Format OK_32", "S3 Format NG_33", "S3 燒入程式 此站執行_34", "S3 燒入程式 OK_35", "S3 燒入程式 NG_36", "S3 備用_37", "S3 備用_38", "S3 動作完成_39", "S4 PC動作中_40", "S4 量測完成 產品正常_41", "S4 量測完成 產品NG_42", "S4 Format 此站執行_43", "S4 Format OK_44", "S4 Format NG_45", "S4 燒入 此站不執行_46", "S4 燒入程式 OK_47", "S4 燒入程式 NG_48", "S4 藍芽Scan OK_49", "S4 藍芽Scan NG_50", "S4 動作完成_51", "給PLC要量電流訊號", "給PLC要量電壓訊號"]
                n339 = flat-sequence {
                  tunnel: [w677] -> w666
                  tunnel: w669 -> [_]
                  frame #0 {
                    n340 = global read "Main Glb.vi" "Discrete Inputs"() -> (w679:bool[])
                    n341 = Index Array(array=w679, index=S2_Station_Input."22_PLC下達可測電壓訊號" ("Enum")) -> (element=w677:bool)
                  }
                }
                n342 = call "Set OutputPLC.vi"("Address In"=20, "Array 2"=w668, "Sat Coils"=bool[] [TRUE]) -> ("Error Out"=w669:errorcluster[])  [unwired: 7 in]
                n343 = case shown="True" w666 {
                  tunnel: [0 w716] -> w675
                  tunnel: w674 -> [w687 w715]
                  tunnel: [w687 w714] -> w673
                  tunnel: w672 -> [_ w713]
                  tunnel: w671 -> [_ w712]
                  tunnel: [errorcluster {"status"=FALSE, "code"=0, "source"=""} ("error IO") w688] -> w670
                  frame False {
                    n344 = call "Auto Inspection_Status.vi"("Action"=enum16{"Initial", "Write", "Read"}."Write", "DataIn"="等待PLC可量壓訊號", "Station"=Auto_Inspection_Station_Name2."S3Measure", "Data"=Auto_Inspection_Data_Name."CurrentAction") -> ()  [unwired: 9 in, 3 out]
                    n345 = Wait (ms)(milliseconds to wait=u32 250) -> ()  [unwired: 1 out]
                  }
                  frame True {
                    w720 = u16 3 items=["SYSTem:VERSion?", "SYSTem:ERRor?", "*IDN?", "MEAS:CURR:DC?", "MEAS:VOLT?", "SYSTem:ERRor?"] ("Ringfor34450A")
                    w719 = u16 5 items=["SYSTem:VERSion?", "SYSTem:ERRor?", "*IDN?", "MEAS:CURR:DC?", "MEAS:VOLT?", "MEAS:VOLT:DC?"] ("RingforIT8511")
                    w717 = u16 0 items=["IT8511", "34450A", "WRBuff"] ("ChangeStatus")
                    # "收尋S2站條碼"
                    # "量電壓"
                    # "T2  T8511A/COM11"
                    n346 = call "Retry Num.vi"("String"=w713) -> ("Numeric"=w726:i32, "retry次數"=w725:string[])  [unwired: 9 in]
                    n347 = call "Auto Inspection_Status.vi"("Action"=enum16{"Initial", "Write", "Read"}."Write", "DataIn"="儀器測量中", "Station"=Auto_Inspection_Station_Name2."S2Measure", "Data"=Auto_Inspection_Data_Name."CurrentAction") -> ()  [unwired: 9 in, 3 out]
                    n348 = local write "retry次數"(w725) -> ()
                    n349 = local write "Retry"(w726) -> ()
                    n350 = call "MTool34450A.vi"("Ringfor34450A"=w720, "RingforIT8511"=w719, "VISA resource name"=refnum<visa-resource-name> "COM11", "ChangeStatus"=w717) -> ("error out"=w721:errorcluster, "μA"=w706:dbl, "read buffer"=w692:string)  [unwired: 4 in, 1 out]
                    "T2 buffer" <- w692
                    "T2 μA" <- w706
                    n351 = Unbundle By Name(w721) -> ("status"=w723:bool)
                    n352 = Number To Fractional String(number=w706) -> (F-format string=w705:string)  [unwired: 3 in]
                    n353 = Increment(x=w712) -> (x+1=w711:i32)
                    n354 = call "AL量測值轉換.vi"("位數"=6, "input string"=w705, "PLC address"=20) -> ("error out"=w708:errorcluster)  [unwired: 7 in, 1 out]
                    n355 = Select(t=w711, s=w723, f=w711) -> (s? t:f=w724:i32)
                    n356 = Not(x=w723) -> (.not. x?=w691:bool)
                    n357 = Greater Or Equal?(x=w724, y=w726) -> (x >= y?=w722:bool)
                    n358 = Increment(x=w715) -> (x+1=w727:i32)
                    n359 = case shown="True" w722 {
                      tunnel: [errorcluster {"status"=FALSE, "code"=0, "source"=""} ("error constant") errorcluster {"status"=TRUE, "code"=18306, "source"=""} ("error constant")] -> w707
                      tunnel: w724 -> [w744 _]
                      tunnel: [w744 0] -> w716
                      tunnel: w721 -> [_ _]
                      frame False {
                      }
                      frame True {
                      }
                    }
                    n360 = disable-structure shown="Disabled" {
                      disable-tunnel: w691 -> [w737 _]
                      disable-tunnel: [w736 _] -> w690
                      frame Disabled {
                        n361 = case shown="True" w737 {
                          tunnel: [w738 w741] -> w736
                          frame False {
                            w740 = T9[] [enum."S4 量測完成 產品NG_42"] items=["S2站PC動作中_20", "電流量測完成產品OK_21", "電流量測完成產品NG_22", "S2站Format 執行_23", "S2 Format OK_24", "S2 Format NG_25", "S2站燒入執行_26", "S2站燒入OK_27", "S2站燒入NG_28", "S2站動作完成_29", "S3 PC動作中_30", "S3 Format 此站執行_31", "S3 Format OK_32", "S3 Format NG_33", "S3 燒入程式 此站執行_34", "S3 燒入程式 OK_35", "S3 燒入程式 NG_36", "S3 備用_37", "S3 備用_38", "S3 動作完成_39", "S4 PC動作中_40", "S4 量測完成 產品正常_41", "S4 量測完成 產品NG_42", "S4 Format 此站執行_43", "S4 Format OK_44", "S4 Format NG_45", "S4 燒入 此站不執行_46", "S4 燒入程式 OK_47", "S4 燒入程式 NG_48", "S4 藍芽Scan OK_49", "S4 藍芽Scan NG_50", "S4 動作完成_51", "給PLC要量電流訊號", "給PLC要量電壓訊號"]
                            n362 = call "Set OutputPLC.vi"("Array"=w740, "Address In"=20) -> ("Error Out"=w738:errorcluster[])  [unwired: 9 in]
                          }
                          frame True {
                            w742 = T9[] [enum."S4 量測完成 產品正常_41"] items=["S2站PC動作中_20", "電流量測完成產品OK_21", "電流量測完成產品NG_22", "S2站Format 執行_23", "S2 Format OK_24", "S2 Format NG_25", "S2站燒入執行_26", "S2站燒入OK_27", "S2站燒入NG_28", "S2站動作完成_29", "S3 PC動作中_30", "S3 Format 此站執行_31", "S3 Format OK_32", "S3 Format NG_33", "S3 燒入程式 此站執行_34", "S3 燒入程式 OK_35", "S3 燒入程式 NG_36", "S3 備用_37", "S3 備用_38", "S3 動作完成_39", "S4 PC動作中_40", "S4 量測完成 產品正常_41", "S4 量測完成 產品NG_42", "S4 Format 此站執行_43", "S4 Format OK_44", "S4 Format NG_45", "S4 燒入 此站不執行_46", "S4 燒入程式 OK_47", "S4 燒入程式 NG_48", "S4 藍芽Scan OK_49", "S4 藍芽Scan NG_50", "S4 動作完成_51", "給PLC要量電流訊號", "給PLC要量電壓訊號"]
                            n363 = call "Set OutputPLC.vi"("Array"=w742, "Address In"=20) -> ("Error Out"=w741:errorcluster[])  [unwired: 9 in]
                          }
                        }
                      }
                      frame Enabled {
                      }
                    }
                    n364 = Select(t=w692, s=w691, f="NG" ("DataIn")) -> (s? t:f=w700:string)
                    n365 = Select(t=w727, s=w691, f=w715) -> (s? t:f=w714:i32)
                    n366 = global read "Main Glb.vi" "Input Registers0-99"() -> (w693:u16[])
                    n367 = Merge Errors(w708, w707) -> (w689:errorcluster)
                    n368 = call "Red PLC InReg.vi"("length"=10, "index"=30, "Input Registers Arr"=w693) -> ("Rad In Reg"=w694:string)  [unwired: 7 in, 1 out]
                    n369 = call "Cub Meaasure FGV.vi"("Action"=Table_Save."Write" ("Enum"), "Save Index"=MeasureDisplayTab."電池負載電壓", "DataIn"=w700, "SN"=w694) -> ()  [unwired: 8 in, 8 out]
                    n370 = Merge Errors(w690, w689) -> (w688:errorcluster)
                    n371 = case shown="Error .." w688 {
                      frame No Error {
                        n372 = global read "Process Global.vi" "S3Tool Action"() -> (w729:bool[])
                        n373 = Replace Array Subset(array=w729, new element=TRUE ("new element/subarray"), index=5) -> (w728:bool[])
                        n374 = global write "Process Global.vi" "S3Tool Action"(w728) -> ()
                      }
                      frame Error {
                        n375 = global read "Process Global.vi" "S3Tool Action"() -> (w735:bool[])
                        n376 = Replace Array Subset(array=w735, new element=FALSE ("new element/subarray"), index=5) -> (w734:bool[])
                        n377 = global write "Process Global.vi" "S3Tool Action"(w734) -> ()
                      }
                    }
                  }
                }
              }
            }
          }
          frame True {
          }
        }
        n378 = property class="DigNum (strict)"(reference=w25, "Value"=w26) -> ()  [unwired: 1 in, 2 out]
        n379 = case shown="Error .." w19 {
          frame No Error {
            n380 = global write "Process Global.vi" "S3 OK"(TRUE) -> ()
          }
          frame Error {
            n381 = global write "Process Global.vi" "S3 NG"(TRUE) -> ()
          }
        }
        n382 = disable-structure shown="Enabled" {
          disable-tunnel: w19 -> [w48 w51]
          disable-tunnel: [w47 w51] -> w20
          frame Disabled {
            n383 = call "ErrorCycleNoSet.vi"("error in"=w48, "CaseNo"=enum16{"S2", "S3", "S4", "S11"}."S3", "Error Set Item"="$AlarmCycleNo_S3") -> ("error out"=w47:errorcluster)  [unwired: 8 in]
          }
          frame Enabled {
          }
        }
        n384 = call "Exit.vi"("Enum"=enum16{"Initial", "Read", "Write"}."Read") -> ("ExitOut"=w22:bool)  [unwired: 10 in]
        n385 = Compound Arithmetic op=OR(w19, w31, w22) -> (w42:bool)
        "present" <- w30
      }
    }
    frame Error {
    }
  }
  n386 = disable-structure shown="Disabled" {
    frame Disabled {
      n387 = global read "Main Glb.vi" "S3 Barcode ID"() -> ()  [unwired: 1 in]
      n388 = global read "Main Glb.vi" "S3 Tary ID"() -> ()  [unwired: 1 in]
    }
    frame Enabled {
    }
  }
  n389 = call "ErrorCycleNoSet.vi"("error in"=w2, "CaseNo"=enum16{"S2", "S3", "S4", "S11"}."S3", "Error Set Item"="$AlarmCycleNo_S3") -> ("error out"=w1:errorcluster)  [unwired: 8 in]
  "error out" <- w1
  n390 = disable-structure shown="Disabled" {
    disable-tunnel: w1 -> [w753 _]
    frame Disabled {
      n391 = case shown="Error .." w753 {
        frame No Error {
          n392 = global write "Process Global.vi" "S3 OK"(TRUE) -> ()
        }
        frame Error {
          n393 = global write "Process Global.vi" "S3 NG"(TRUE) -> ()
        }
      }
    }
    frame Enabled {
    }
  }
  n394 = Select(t=Station_Action."Dectect Action" ("Station Out"), s=w1, f=Station_Action."ImformOut" ("Station Out")) -> (s? t:f=→"Station Out":T1)
  "AI out" <- "AI in"
